vi "Q2_TorresHan.vi"() -> ()   [LabVIEW 2020]
uses:
  <vilib>/Utility/miscctls.llb/LVPoint32TypeDef.ctl
  <vilib>/Utility/miscctls.llb/LVPositionTypeDef.ctl
  <vilib>/Utility/miscctls.llb/LVBoundsTypeDef.ctl
  <vilib>/Utility/inputDevices.llb/mouseAcquire.vi
  <vilib>/Utility/inputDevices.llb/closeMouse.vi
panel:
  in  "instrucciones":bool
  out "pasos":string
  out "mensaje":string
  in  "Iniciar":bool
  out "estado":u16
  out "discoaMover":string
  out "positionIncialTorre":i32
  out "evento":u32
  out "positionIncialDisco":T1
  out "referenciaDisco":refnum<vi>
  out "mouseActivoPorEvento?":bool=TRUE
  out "mouse":bool
  out "coordenadas del mouse":T2
  out "Tu numero de movimientos":i16
  out "Minimos de movimientos":u16
  in  "Numero de discos":enum16{"3", "4", "5"}(ring)
  out "5":bool
  out "4":bool
  out "3":bool
  out "2":bool
  out "1":bool
  out "disco5 4":bool
  out "disco5 3":bool
  out "disco5 2":bool
  out "BASE":bool
  out "TORRE2":bool
  out "TORRE3":bool
  out "TORRE1":bool
  # "TORRE 1"
  # "TORRE 2"
  # "TORRE 3"
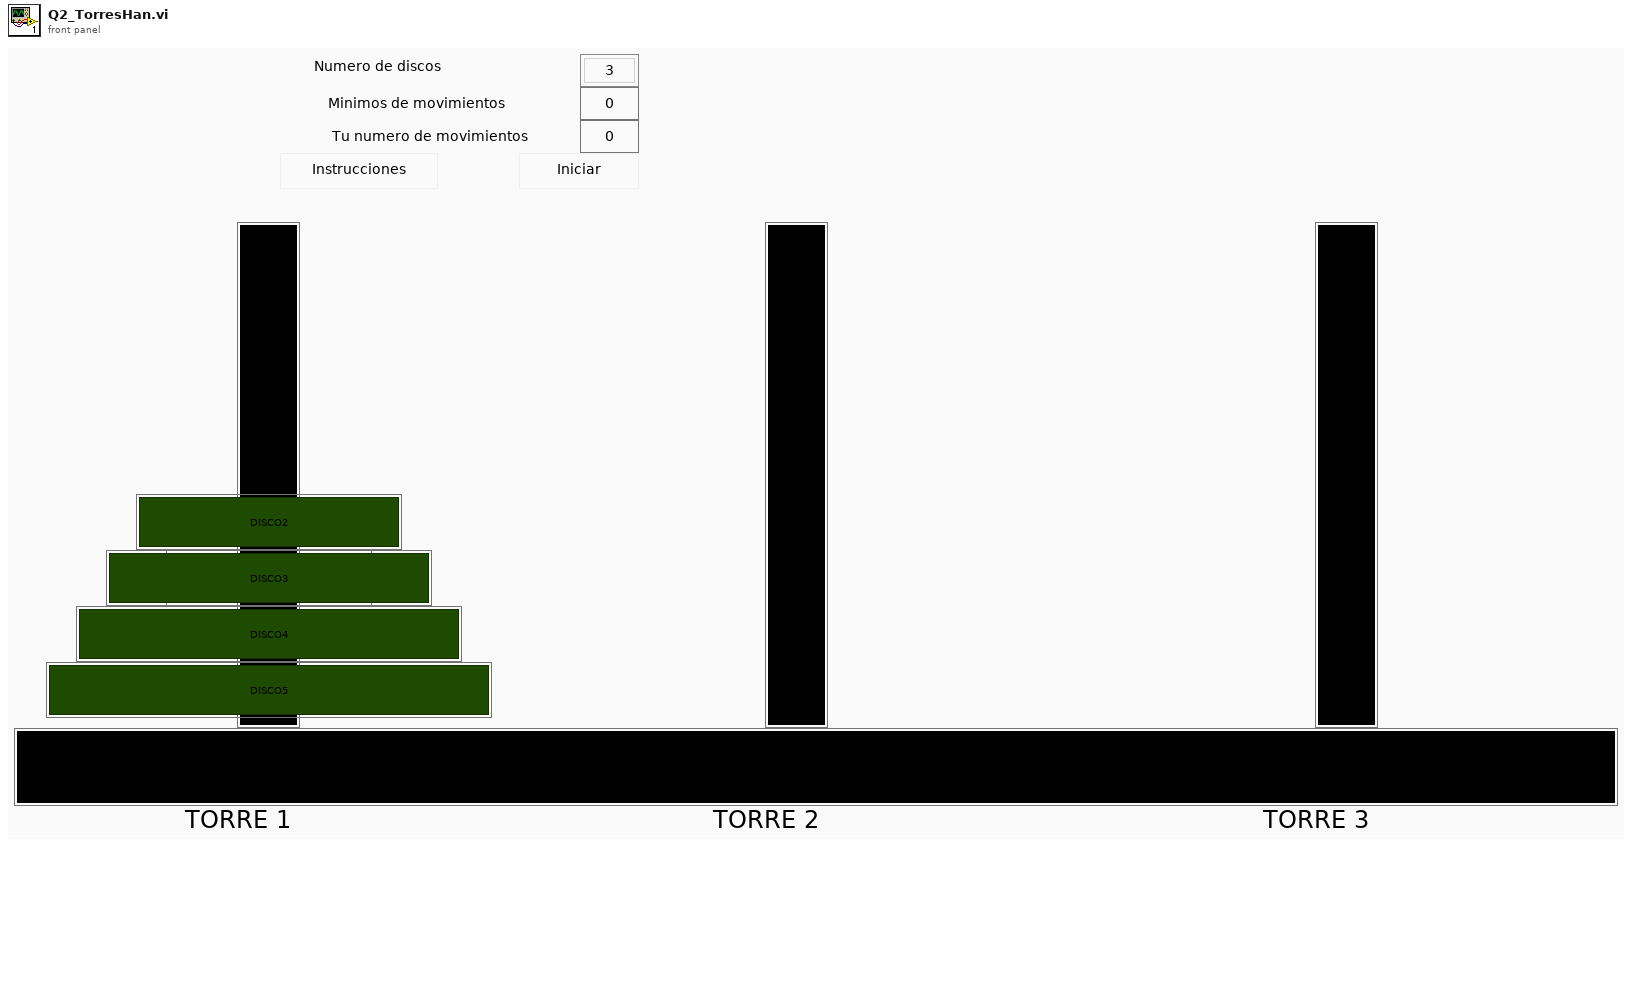
[diagram p1: front panel]
types:
  T1 = typedef "LVPositionTypeDef.ctl" = cluster{"Left":i32, "Top":i32}
  T2 = typedef "LVPoint32TypeDef.ctl" = cluster{"Horizontal":i32, "Vertical":i32}
  T3 = typedef "LVBoundsTypeDef.ctl" = cluster{"Width":u32, "Height":u32}
  T4 = cluster{"button 1":bool, "button 2":bool, "button 3":bool, "button 4":bool}
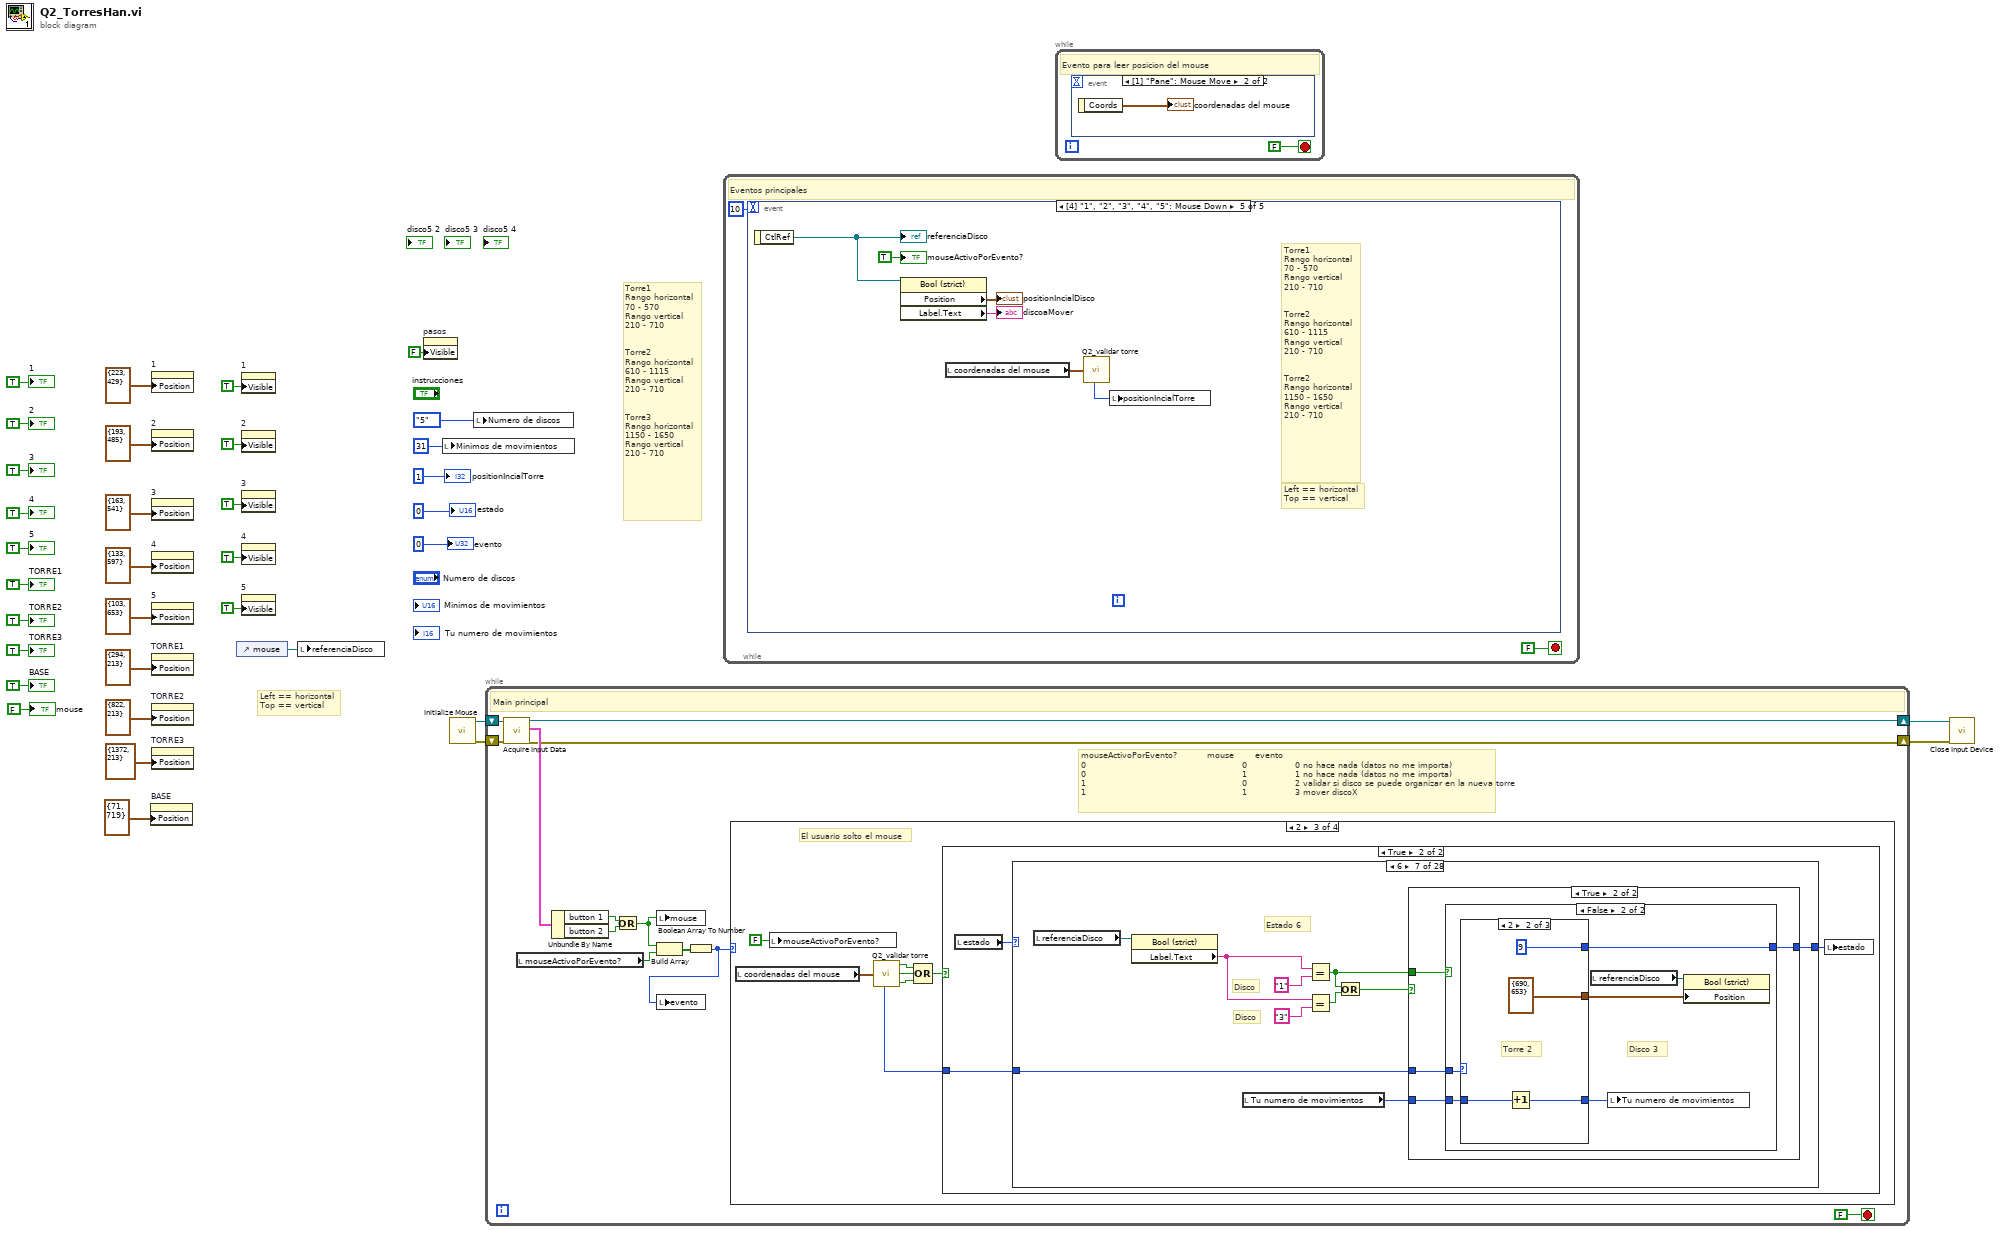
[diagram p0: block diagram]
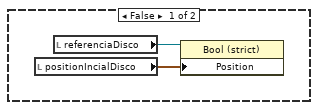
[diagram p4: hidden frame]
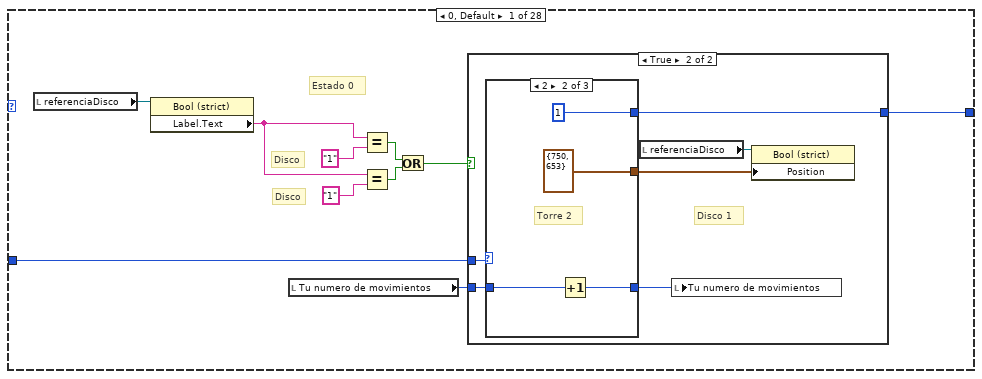
[diagram p5: hidden frame]
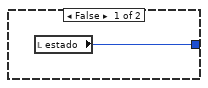
[diagram p6: hidden frame]
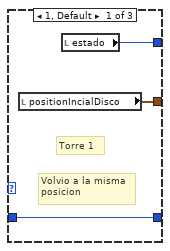
[diagram p7: hidden frame]
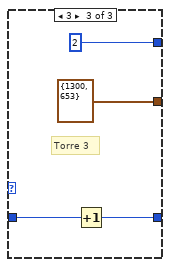
[diagram p8: hidden frame]
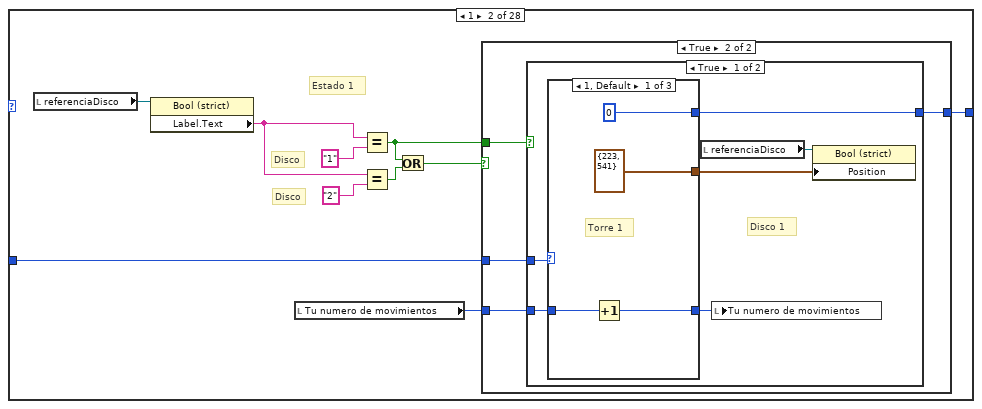
[diagram p9: hidden frame]
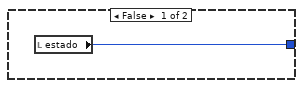
[diagram p10: hidden frame]
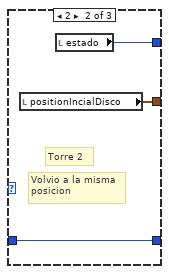
[diagram p11: hidden frame]
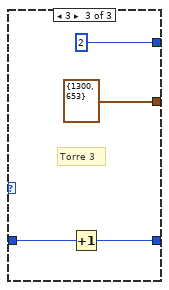
[diagram p12: hidden frame]
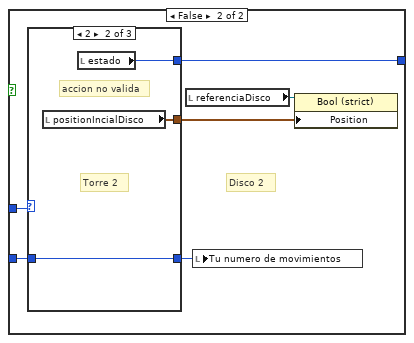
[diagram p13: hidden frame]
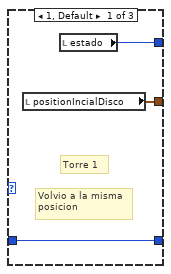
[diagram p14: hidden frame]
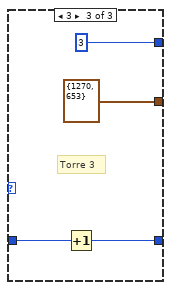
[diagram p15: hidden frame]
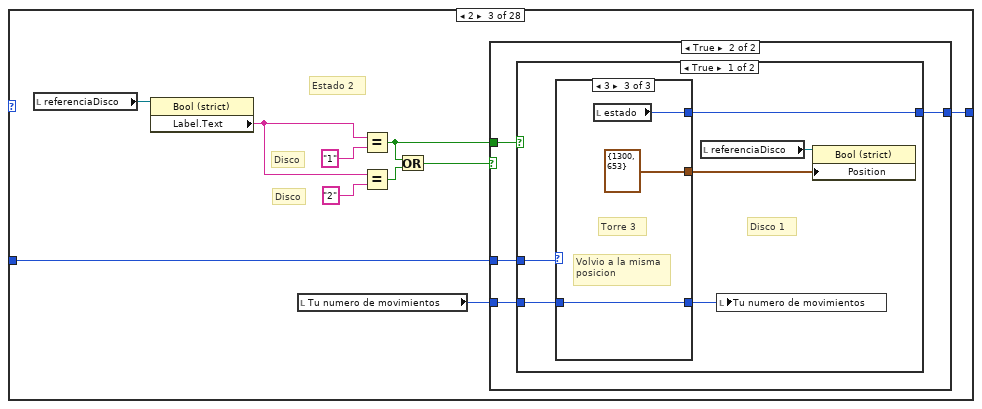
[diagram p16: hidden frame]
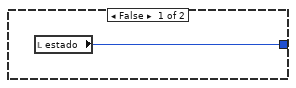
[diagram p17: hidden frame]
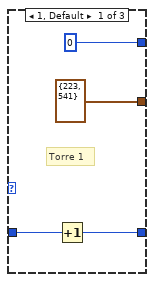
[diagram p18: hidden frame]
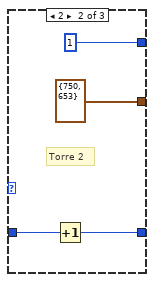
[diagram p19: hidden frame]
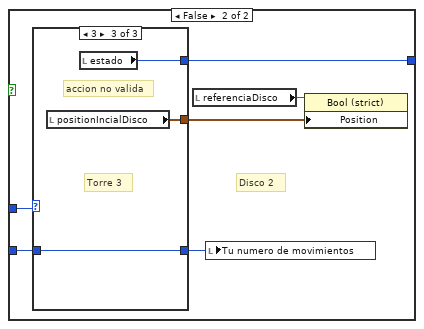
[diagram p20: hidden frame]
diagram:
  # "Left == horizontal\nTop == vertical"
  # "Torre1\nRango horizontal\n70 - 570\nRango vertical\n210 - 710\n\n\nTorre2\nRango horizontal\n610 - 1115\nRango vertical\n210 - 710\n\n\nTorre3\nRango horizontal\n1150 - 1650\nRango vertical\n210 - 710"
  n1 = property on="BASE" class="Bool (strict)"("Position"=T1 {"Left"=71, "Top"=719}) -> ()  [unwired: 2 in, 2 out]
  n2 = property on="1" class="Bool (strict)"("Position"=T1 {"Left"=223, "Top"=429}) -> ()  [unwired: 2 in, 2 out]
  n3 = property on="2" class="Bool (strict)"("Position"=T1 {"Left"=193, "Top"=485}) -> ()  [unwired: 2 in, 2 out]
  n4 = property on="3" class="Bool (strict)"("Position"=T1 {"Left"=163, "Top"=541}) -> ()  [unwired: 2 in, 2 out]
  n5 = property on="4" class="Bool (strict)"("Position"=T1 {"Left"=133, "Top"=597}) -> ()  [unwired: 2 in, 2 out]
  n6 = property on="5" class="Bool (strict)"("Position"=T1 {"Left"=103, "Top"=653}) -> ()  [unwired: 2 in, 2 out]
  n7 = property on="TORRE1" class="Bool (strict)"("Position"=T1 {"Left"=294, "Top"=213}) -> ()  [unwired: 2 in, 2 out]
  n8 = property on="TORRE2" class="Bool (strict)"("Position"=T1 {"Left"=822, "Top"=213}) -> ()  [unwired: 2 in, 2 out]
  n9 = property on="TORRE3" class="Bool (strict)"("Position"=T1 {"Left"=1372, "Top"=213}) -> ()  [unwired: 2 in, 2 out]
  n10 = control-ref of="mouse"() -> (w2:refnum<vi>)
  n11 = property on="1" class="Bool (strict)"("Visible"=TRUE) -> ()  [unwired: 2 in, 2 out]
  n12 = property on="2" class="Bool (strict)"("Visible"=TRUE) -> ()  [unwired: 2 in, 2 out]
  n13 = property on="3" class="Bool (strict)"("Visible"=TRUE) -> ()  [unwired: 2 in, 2 out]
  n14 = property on="4" class="Bool (strict)"("Visible"=TRUE) -> ()  [unwired: 2 in, 2 out]
  n15 = property on="5" class="Bool (strict)"("Visible"=TRUE) -> ()  [unwired: 2 in, 2 out]
  n16 = local write "referenciaDisco"(w2) -> ()
  n17 = property on="pasos" class="Str"("Visible"=FALSE) -> ()  [unwired: 2 in, 2 out]
  n18 = local write "Minimos de movimientos"(u16 31 ("Minimos de movimientos")) -> ()
  n19 = call <vilib>:"Initialize Mouse.vi"() -> ("error out"=w5:errorcluster, "device ID"=w6:refnum<k1>)  [unwired: 10 in]
  n20 = local write "Numero de discos"(enum16{"3", "4", "5"}."5" ("Numero de discos")) -> ()
  n21 = while {
    shift-right: [w44] -> w4
    shift-left: w6 -> [w46]
    shift-right: [w43] -> w3
    shift-left: w5 -> [w45]
    stop <- FALSE stop-if-true
    # "mouseActivoPorEvento?\t         mouse\t      evento\n0\t\t                                                  0\t               0 no hace nada (datos no me importa)\n0\t\t                                                  1\t               1 no hace nada (datos no me importa)\n1\t\t                                                  0\t               2 validar si disco se puede organizar en la nueva torre\n1\t\t                                                  1\t               3 mover discoX"
    # "Main principal"
    n22 = call-poly <vilib>:"Acquire Input Data.vi"("device ID"=w46, "error in (no error)"=w45) -> ("device ID"=w44:refnum<k1>, "button info"=w47:T4, "error out"=w43:errorcluster)  [unwired: 14 in, 1 out]
    n23 = local read "mouseActivoPorEvento?"() -> (w40:bool)
    n24 = Unbundle By Name(w47) -> ("button 1"=w42:bool, "button 2"=w41:bool)
    n25 = Or(x=w42, y=w41) -> (x .or. y?=w38:bool)
    n26 = local write "mouse"(w38) -> ()
    n27 = Build Array(w38, w40) -> (w39:bool[])
    n28 = Boolean Array To Number(Boolean array=w39) -> (number=w37:u32)
    n29 = local write "evento"(w37) -> ()
    n30 = case shown="2" w37 {
      frame 0, Default {
      }
      frame 1 {
      }
      frame 2 {
        # "El usuario solto el mouse"
        n31 = local read "coordenadas del mouse"() -> (w54:T2)
        n32 = local write "mouseActivoPorEvento?"(FALSE ("mouseActivoPorEvento?")) -> ()
        n33 = call "Q2_validar torre.vi"("coordenadas del mouse"=w54) -> ("Torre"=w48:i32, "torre1"=w51:bool, "torre2"=w52:bool, "torre3"=w53:bool)  [unwired: 3 in]
        n34 = Compound Arithmetic op=OR(w51, w52, w53) -> (w49:bool)
        n35 = case shown="True" w49 {
          tunnel: w48 -> [_ w59]
          frame False {
            n36 = local read "positionIncialDisco"() -> (w56:T1)
            n37 = local read "referenciaDisco"() -> (w55:refnum<vi>)
            n38 = property class="Bool (strict)"(reference=w55, "Position"=w56) -> ()  [unwired: 1 in, 2 out]
          }
          frame True {
            n39 = local read "estado"() -> (w58:u16)
            n40 = case shown="6" w58 {
              tunnel: w59 -> [w69 w97 w145 w193 w241 w289 w337 w385 w433 w481 w529 w577 w625 w673 w721 w769 w817 w865 w913 w961 w1009 w1037 w1085 w1133 w1181 w1229 w1257 w1305]
              tunnel: [w68 w96 w144 w192 w240 w288 w336 w384 w432 w480 w528 w576 w624 w672 w720 w768 w816 w864 w912 w960 w1008 w1036 w1084 w1132 w1180 w1228 w1256 w1304] -> w57
              frame 0, Default {
                # "Disco"
                # "Disco"
                # "Estado 0"
                n41 = local read "referenciaDisco"() -> (w64:refnum<vi>)
                n42 = property class="Bool (strict)"(reference=w64) -> ("Label.Text"=w65:string)  [unwired: 1 in, 2 out]
                n43 = local read "Tu numero de movimientos"() -> (w60:i16)
                n44 = Equal?(x=w65, y="1") -> (x = y?=w67:bool)
                n45 = Equal?(x=w65, y="1") -> (x = y?=w66:bool)
                n46 = Or(x=w67, y=w66) -> (x .or. y?=w61:bool)
                n47 = case shown="True" w61 {
                  tunnel: w69 -> [_ w75]
                  tunnel: [w70 w73] -> w68
                  tunnel: w60 -> [_ w71]
                  frame False {
                    n48 = local read "estado"() -> (w70:u16)
                  }
                  frame True {
                    # "Disco 1"
                    n49 = case shown="2" w75 {
                      tunnel: [w79 T1 {"Left"=750, "Top"=653} ("Position") T1 {"Left"=1300, "Top"=653} ("Position")] -> w74
                      tunnel: [w77 u16 1 ("estado") u16 2 ("estado")] -> w73
                      tunnel: [w78 w80 w84] -> w72
                      tunnel: w71 -> [w78 w81 w85]
                      frame 1, Default {
                        # "Volvio a la misma\nposicion"
                        # "Torre 1"
                        n50 = local read "positionIncialDisco"() -> (w79:T1)
                        n51 = local read "estado"() -> (w77:u16)
                      }
                      frame 2 {
                        # "Torre 2"
                        n52 = Increment(x=w81) -> (x+1=w80:i16)
                      }
                      frame 3 {
                        # "Torre 3"
                        n53 = Increment(x=w85) -> (x+1=w84:i16)
                      }
                    }
                    n54 = local read "referenciaDisco"() -> (w76:refnum<vi>)
                    n55 = local write "Tu numero de movimientos"(w72) -> ()
                    n56 = property class="Bool (strict)"(reference=w76, "Position"=w74) -> ()  [unwired: 1 in, 2 out]
                  }
                }
              }
              frame 1 {
                # "Disco"
                # "Disco"
                # "Estado 1"
                n57 = local read "referenciaDisco"() -> (w93:refnum<vi>)
                n58 = property class="Bool (strict)"(reference=w93) -> ("Label.Text"=w94:string)  [unwired: 1 in, 2 out]
                n59 = local read "Tu numero de movimientos"() -> (w88:i16)
                n60 = Equal?(x=w94, y="1") -> (x = y?=w89:bool)
                n61 = Equal?(x=w94, y="2") -> (x = y?=w95:bool)
                n62 = Or(x=w89, y=w95) -> (x .or. y?=w90:bool)
                n63 = case shown="True" w90 {
                  tunnel: w97 -> [_ w102]
                  tunnel: [w98 w101] -> w96
                  tunnel: w89 -> [_ w100]
                  tunnel: w88 -> [_ w99]
                  frame False {
                    n64 = local read "estado"() -> (w98:u16)
                  }
                  frame True {
                    n65 = case shown="True" w100 {
                      tunnel: w102 -> [w107 w124]
                      tunnel: [w105 w122] -> w101
                      tunnel: w99 -> [w103 w120]
                      frame True {
                        # "Disco 1"
                        n66 = case shown="1, Default" w107 {
                          tunnel: [T1 {"Left"=223, "Top"=541} ("Position") w114 T1 {"Left"=1300, "Top"=653} ("Position")] -> w106
                          tunnel: [u16 0 ("estado") w113 u16 2 ("estado")] -> w105
                          tunnel: [w109 w115 w116] -> w104
                          tunnel: w103 -> [w110 w115 w117]
                          frame 1, Default {
                            # "Torre 1"
                            n67 = Increment(x=w110) -> (x+1=w109:i16)
                          }
                          frame 2 {
                            # "Volvio a la misma\nposicion"
                            # "Torre 2"
                            n68 = local read "positionIncialDisco"() -> (w114:T1)
                            n69 = local read "estado"() -> (w113:u16)
                          }
                          frame 3 {
                            # "Torre 3"
                            n70 = Increment(x=w117) -> (x+1=w116:i16)
                          }
                        }
                        n71 = local read "referenciaDisco"() -> (w108:refnum<vi>)
                        n72 = local write "Tu numero de movimientos"(w104) -> ()
                        n73 = property class="Bool (strict)"(reference=w108, "Position"=w106) -> ()  [unwired: 1 in, 2 out]
                      }
                      frame False {
                        # "Disco 2"
                        n74 = case shown="2" w124 {
                          tunnel: [w128 w131 T1 {"Left"=1270, "Top"=653} ("Position")] -> w123
                          tunnel: [w126 w129 u16 3 ("estado")] -> w122
                          tunnel: [w127 w130 w132] -> w121
                          tunnel: w120 -> [w127 w130 w133]
                          frame 1, Default {
                            # "Volvio a la misma\nposicion"
                            # "Torre 1"
                            n75 = local read "positionIncialDisco"() -> (w128:T1)
                            n76 = local read "estado"() -> (w126:u16)
                          }
                          frame 2 {
                            # "accion no valida"
                            # "Torre 2"
                            n77 = local read "positionIncialDisco"() -> (w131:T1)
                            n78 = local read "estado"() -> (w129:u16)
                          }
                          frame 3 {
                            # "Torre 3"
                            n79 = Increment(x=w133) -> (x+1=w132:i16)
                          }
                        }
                        n80 = local read "referenciaDisco"() -> (w125:refnum<vi>)
                        n81 = local write "Tu numero de movimientos"(w121) -> ()
                        n82 = property class="Bool (strict)"(reference=w125, "Position"=w123) -> ()  [unwired: 1 in, 2 out]
                      }
                    }
                  }
                }
              }
              frame 2 {
                # "Disco"
                # "Disco"
                # "Estado 2"
                n83 = local read "referenciaDisco"() -> (w141:refnum<vi>)
                n84 = property class="Bool (strict)"(reference=w141) -> ("Label.Text"=w142:string)  [unwired: 1 in, 2 out]
                n85 = local read "Tu numero de movimientos"() -> (w136:i16)
                n86 = Equal?(x=w142, y="1") -> (x = y?=w137:bool)
                n87 = Equal?(x=w142, y="2") -> (x = y?=w143:bool)
                n88 = Or(x=w137, y=w143) -> (x .or. y?=w138:bool)
                n89 = case shown="True" w138 {
                  tunnel: w145 -> [_ w150]
                  tunnel: [w146 w149] -> w144
                  tunnel: w137 -> [_ w148]
                  tunnel: w136 -> [_ w147]
                  frame False {
                    n90 = local read "estado"() -> (w146:u16)
                  }
                  frame True {
                    n91 = case shown="True" w148 {
                      tunnel: w150 -> [w155 w172]
                      tunnel: [w153 w170] -> w149
                      tunnel: w147 -> [w151 w168]
                      frame True {
                        # "Disco 1"
                        n92 = case shown="3" w155 {
                          tunnel: [T1 {"Left"=223, "Top"=541} ("Position") T1 {"Left"=750, "Top"=653} ("Position") T1 {"Left"=1300, "Top"=653} ("Position")] -> w154
                          tunnel: [u16 0 ("estado") u16 1 ("estado") w165] -> w153
                          tunnel: [w157 w161 w166] -> w152
                          tunnel: w151 -> [w158 w162 w166]
                          frame 1, Default {
                            # "Torre 1"
                            n93 = Increment(x=w158) -> (x+1=w157:i16)
                          }
                          frame 2 {
                            # "Torre 2"
                            n94 = Increment(x=w162) -> (x+1=w161:i16)
                          }
                          frame 3 {
                            # "Volvio a la misma\nposicion"
                            # "Torre 3"
                            n95 = local read "estado"() -> (w165:u16)
                          }
                        }
                        n96 = local read "referenciaDisco"() -> (w156:refnum<vi>)
                        n97 = local write "Tu numero de movimientos"(w152) -> ()
                        n98 = property class="Bool (strict)"(reference=w156, "Position"=w154) -> ()  [unwired: 1 in, 2 out]
                      }
                      frame False {
                        # "Disco 2"
                        n99 = case shown="3" w172 {
                          tunnel: [w176 T1 {"Left"=720, "Top"=653} ("Position") w183] -> w171
                          tunnel: [w174 u16 4 ("estado") w181] -> w170
                          tunnel: [w175 w177 w182] -> w169
                          tunnel: w168 -> [w175 w178 w182]
                          frame 1, Default {
                            # "Volvio a la misma\nposicion"
                            # "Torre 1"
                            n100 = local read "positionIncialDisco"() -> (w176:T1)
                            n101 = local read "estado"() -> (w174:u16)
                          }
                          frame 2 {
                            # "Torre 2"
                            n102 = Increment(x=w178) -> (x+1=w177:i16)
                          }
                          frame 3 {
                            # "accion no valida"
                            # "Torre 3"
                            n103 = local read "positionIncialDisco"() -> (w183:T1)
                            n104 = local read "estado"() -> (w181:u16)
                          }
                        }
                        n105 = local read "referenciaDisco"() -> (w173:refnum<vi>)
                        n106 = local write "Tu numero de movimientos"(w169) -> ()
                        n107 = property class="Bool (strict)"(reference=w173, "Position"=w171) -> ()  [unwired: 1 in, 2 out]
                      }
                    }
                  }
                }
              }
              frame 3 {
                # "Disco"
                # "Disco"
                # "Estado 3"
                n108 = local read "referenciaDisco"() -> (w189:refnum<vi>)
                n109 = property class="Bool (strict)"(reference=w189) -> ("Label.Text"=w190:string)  [unwired: 1 in, 2 out]
                n110 = local read "Tu numero de movimientos"() -> (w184:i16)
                n111 = Equal?(x=w190, y="1") -> (x = y?=w185:bool)
                n112 = Equal?(x=w190, y="2") -> (x = y?=w191:bool)
                n113 = Or(x=w185, y=w191) -> (x .or. y?=w186:bool)
                n114 = case shown="True" w186 {
                  tunnel: w193 -> [_ w198]
                  tunnel: [w194 w197] -> w192
                  tunnel: w185 -> [_ w196]
                  tunnel: w184 -> [_ w195]
                  frame False {
                    n115 = local read "estado"() -> (w194:u16)
                  }
                  frame True {
                    n116 = case shown="True" w196 {
                      tunnel: w198 -> [w203 w220]
                      tunnel: [w201 w218] -> w197
                      tunnel: w195 -> [w199 w216]
                      frame True {
                        # "Disco 1"
                        n117 = case shown="3" w203 {
                          tunnel: [T1 {"Left"=223, "Top"=597} ("Position") w211 T1 {"Left"=1300, "Top"=597} ("Position")] -> w202
                          tunnel: [u16 5 ("estado") w210 u16 6 ("estado")] -> w201
                          tunnel: [w205 w209 w212] -> w200
                          tunnel: w199 -> [w206 w209 w213]
                          frame 1, Default {
                            # "Torre 1"
                            n118 = Increment(x=w206) -> (x+1=w205:i16)
                          }
                          frame 2 {
                            # "Volvio a la misma\nposicion"
                            # "Torre 2"
                            n119 = local read "positionIncialDisco"() -> (w211:T1)
                            n120 = local read "estado"() -> (w210:u16)
                          }
                          frame 3 {
                            # "Torre 3"
                            n121 = Increment(x=w213) -> (x+1=w212:i16)
                          }
                        }
                        n122 = local read "referenciaDisco"() -> (w204:refnum<vi>)
                        n123 = local write "Tu numero de movimientos"(w200) -> ()
                        n124 = property class="Bool (strict)"(reference=w204, "Position"=w202) -> ()  [unwired: 1 in, 2 out]
                      }
                      frame False {
                        # "Disco 2"
                        n125 = case shown="2" w220 {
                          tunnel: [T1 {"Left"=193, "Top"=597} ("Position") w228 w231] -> w219
                          tunnel: [u16 1 ("estado") w226 w230] -> w218
                          tunnel: [w222 w227 w229] -> w217
                          tunnel: w216 -> [w223 w227 w229]
                          frame 1, Default {
                            # "Torre 1"
                            n126 = Increment(x=w223) -> (x+1=w222:i16)
                          }
                          frame 2 {
                            # "accion no valida"
                            # "Torre 2"
                            n127 = local read "positionIncialDisco"() -> (w228:T1)
                            n128 = local read "estado"() -> (w226:u16)
                          }
                          frame 3 {
                            # "Volvio a la misma\nposicion"
                            # "Torre 3"
                            n129 = local read "positionIncialDisco"() -> (w231:T1)
                            n130 = local read "estado"() -> (w230:u16)
                          }
                        }
                        n131 = local read "referenciaDisco"() -> (w221:refnum<vi>)
                        n132 = local write "Tu numero de movimientos"(w217) -> ()
                        n133 = property class="Bool (strict)"(reference=w221, "Position"=w219) -> ()  [unwired: 1 in, 2 out]
                      }
                    }
                  }
                }
              }
              frame 4 {
                # "Disco"
                # "Disco"
                # "Estado 4"
                n134 = local read "referenciaDisco"() -> (w237:refnum<vi>)
                n135 = property class="Bool (strict)"(reference=w237) -> ("Label.Text"=w238:string)  [unwired: 1 in, 2 out]
                n136 = local read "Tu numero de movimientos"() -> (w232:i16)
                n137 = Equal?(x=w238, y="1") -> (x = y?=w233:bool)
                n138 = Equal?(x=w238, y="2") -> (x = y?=w239:bool)
                n139 = Or(x=w233, y=w239) -> (x .or. y?=w234:bool)
                n140 = case shown="True" w234 {
                  tunnel: w241 -> [_ w246]
                  tunnel: [w242 w245] -> w240
                  tunnel: w233 -> [_ w244]
                  tunnel: w232 -> [_ w243]
                  frame False {
                    n141 = local read "estado"() -> (w242:u16)
                  }
                  frame True {
                    n142 = case shown="True" w244 {
                      tunnel: w246 -> [w251 w268]
                      tunnel: [w249 w266] -> w245
                      tunnel: w243 -> [w247 w264]
                      frame True {
                        # "Disco 1"
                        n143 = case shown="2" w251 {
                          tunnel: [T1 {"Left"=223, "Top"=597} ("Position") T1 {"Left"=750, "Top"=597} ("Position") w263] -> w250
                          tunnel: [u16 7 ("estado") u16 8 ("estado") w262] -> w249
                          tunnel: [w253 w257 w261] -> w248
                          tunnel: w247 -> [w254 w258 w261]
                          frame 1, Default {
                            # "Torre 1"
                            n144 = Increment(x=w254) -> (x+1=w253:i16)
                          }
                          frame 2 {
                            # "Torre 2"
                            n145 = Increment(x=w258) -> (x+1=w257:i16)
                          }
                          frame 3 {
                            # "Volvio a la misma\nposicion"
                            # "Torre 3"
                            n146 = local read "positionIncialDisco"() -> (w263:T1)
                            n147 = local read "estado"() -> (w262:u16)
                          }
                        }
                        n148 = local read "referenciaDisco"() -> (w252:refnum<vi>)
                        n149 = local write "Tu numero de movimientos"(w248) -> ()
                        n150 = property class="Bool (strict)"(reference=w252, "Position"=w250) -> ()  [unwired: 1 in, 2 out]
                      }
                      frame False {
                        # "Disco 2"
                        n151 = case shown="3" w268 {
                          tunnel: [T1 {"Left"=193, "Top"=597} ("Position") w276 w279] -> w267
                          tunnel: [u16 2 ("estado") w274 w277] -> w266
                          tunnel: [w270 w275 w278] -> w265
                          tunnel: w264 -> [w271 w275 w278]
                          frame 1, Default {
                            # "Torre 1"
                            n152 = Increment(x=w271) -> (x+1=w270:i16)
                          }
                          frame 2 {
                            # "Volvio a la misma\nposicion"
                            # "Torre 2"
                            n153 = local read "positionIncialDisco"() -> (w276:T1)
                            n154 = local read "estado"() -> (w274:u16)
                          }
                          frame 3 {
                            # "accion no valida"
                            # "Torre 3"
                            n155 = local read "positionIncialDisco"() -> (w279:T1)
                            n156 = local read "estado"() -> (w277:u16)
                          }
                        }
                        n157 = local read "referenciaDisco"() -> (w269:refnum<vi>)
                        n158 = local write "Tu numero de movimientos"(w265) -> ()
                        n159 = property class="Bool (strict)"(reference=w269, "Position"=w267) -> ()  [unwired: 1 in, 2 out]
                      }
                    }
                  }
                }
              }
              frame 5 {
                # "Disco"
                # "Disco"
                # "Estado 5"
                n160 = local read "referenciaDisco"() -> (w285:refnum<vi>)
                n161 = property class="Bool (strict)"(reference=w285) -> ("Label.Text"=w286:string)  [unwired: 1 in, 2 out]
                n162 = local read "Tu numero de movimientos"() -> (w280:i16)
                n163 = Equal?(x=w286, y="1") -> (x = y?=w281:bool)
                n164 = Equal?(x=w286, y="2") -> (x = y?=w287:bool)
                n165 = Or(x=w281, y=w287) -> (x .or. y?=w282:bool)
                n166 = case shown="True" w282 {
                  tunnel: w289 -> [_ w294]
                  tunnel: [w290 w293] -> w288
                  tunnel: w281 -> [_ w292]
                  tunnel: w280 -> [_ w291]
                  frame False {
                    n167 = local read "estado"() -> (w290:u16)
                  }
                  frame True {
                    n168 = case shown="False" w292 {
                      tunnel: w294 -> [w299 w316]
                      tunnel: [w297 w314] -> w293
                      tunnel: w291 -> [w295 w312]
                      frame True {
                        # "Disco 1"
                        n169 = case shown="1, Default" w299 {
                          tunnel: [w301 T1 {"Left"=750, "Top"=653} ("Position") T1 {"Left"=1300, "Top"=597} ("Position")] -> w298
                          tunnel: [w302 u16 3 ("estado") u16 6 ("estado")] -> w297
                          tunnel: [w303 w304 w308] -> w296
                          tunnel: w295 -> [w303 w305 w311]
                          frame 1, Default {
                            # "Volvio a la misma\nposicion"
                            # "Torre 1"
                            n170 = local read "positionIncialDisco"() -> (w301:T1)
                            n171 = local read "estado"() -> (w302:u16)
                          }
                          frame 2 {
                            # "Torre 2"
                            n172 = Increment(x=w305) -> (x+1=w304:i16)
                          }
                          frame 3 {
                            # "Torre 3"
                            n173 = Increment(x=w311) -> (x+1=w308:i16)
                          }
                        }
                        n174 = local read "referenciaDisco"() -> (w300:refnum<vi>)
                        n175 = local write "Tu numero de movimientos"(w296) -> ()
                        n176 = property class="Bool (strict)"(reference=w300, "Position"=w298) -> ()  [unwired: 1 in, 2 out]
                      }
                      frame False {
                        # "Disco 2"
                        n177 = case shown="1, Default" w316 {
                          tunnel: [w319 T1 {"Left"=720, "Top"=653} ("Position") w326] -> w315
                          tunnel: [w318 u16 7 ("estado") w325] -> w314
                          tunnel: [w320 w322 w327] -> w313
                          tunnel: w312 -> [w320 w324 w327]
                          frame 1, Default {
                            # "accion no valida"
                            # "Torre 1"
                            n178 = local read "positionIncialDisco"() -> (w319:T1)
                            n179 = local read "estado"() -> (w318:u16)
                          }
                          frame 2 {
                            # "Torre 2"
                            n180 = Increment(x=w324) -> (x+1=w322:i16)
                          }
                          frame 3 {
                            # "Volvio a la misma\nposicion"
                            # "Torre 3"
                            n181 = local read "positionIncialDisco"() -> (w326:T1)
                            n182 = local read "estado"() -> (w325:u16)
                          }
                        }
                        n183 = local read "referenciaDisco"() -> (w317:refnum<vi>)
                        n184 = local write "Tu numero de movimientos"(w313) -> ()
                        n185 = property class="Bool (strict)"(reference=w317, "Position"=w315) -> ()  [unwired: 1 in, 2 out]
                      }
                    }
                  }
                }
              }
              frame 6 {
                # "Disco"
                # "Disco"
                # "Estado 6"
                n186 = local read "referenciaDisco"() -> (w333:refnum<vi>)
                n187 = property class="Bool (strict)"(reference=w333) -> ("Label.Text"=w334:string)  [unwired: 1 in, 2 out]
                n188 = local read "Tu numero de movimientos"() -> (w328:i16)
                n189 = Equal?(x=w334, y="1") -> (x = y?=w329:bool)
                n190 = Equal?(x=w334, y="3") -> (x = y?=w335:bool)
                n191 = Or(x=w329, y=w335) -> (x .or. y?=w330:bool)
                n192 = case shown="True" w330 {
                  tunnel: w337 -> [_ w342]
                  tunnel: [w338 w341] -> w336
                  tunnel: w329 -> [_ w340]
                  tunnel: w328 -> [_ w339]
                  frame False {
                    n193 = local read "estado"() -> (w338:u16)
                  }
                  frame True {
                    n194 = case shown="False" w340 {
                      tunnel: w342 -> [w347 w364]
                      tunnel: [w345 w362] -> w341
                      tunnel: w339 -> [w343 w360]
                      frame True {
                        # "Disco 1"
                        n195 = case shown="1, Default" w347 {
                          tunnel: [T1 {"Left"=223, "Top"=597} ("Position") T1 {"Left"=750, "Top"=653} ("Position") w357] -> w346
                          tunnel: [u16 5 ("estado") u16 3 ("estado") w358] -> w345
                          tunnel: [w349 w353 w359] -> w344
                          tunnel: w343 -> [w352 w354 w359]
                          frame 1, Default {
                            # "Torre 1"
                            n196 = Increment(x=w352) -> (x+1=w349:i16)
                          }
                          frame 2 {
                            # "Torre 2"
                            n197 = Increment(x=w354) -> (x+1=w353:i16)
                          }
                          frame 3 {
                            # "Volvio a la misma\nposicion"
                            # "Torre 3"
                            n198 = local read "positionIncialDisco"() -> (w357:T1)
                            n199 = local read "estado"() -> (w358:u16)
                          }
                        }
                        n200 = local read "referenciaDisco"() -> (w348:refnum<vi>)
                        n201 = local write "Tu numero de movimientos"(w344) -> ()
                        n202 = property class="Bool (strict)"(reference=w348, "Position"=w346) -> ()  [unwired: 1 in, 2 out]
                      }
                      frame False {
                        # "Disco 3"
                        n203 = case shown="2" w364 {
                          tunnel: [w367 T1 {"Left"=690, "Top"=653} ("Position") w374] -> w363
                          tunnel: [w366 u16 9 ("estado") w373] -> w362
                          tunnel: [w368 w370 w375] -> w361
                          tunnel: w360 -> [w368 w372 w375]
                          frame 1, Default {
                            # "Volvio a la misma\nposicion"
                            # "Torre 1"
                            n204 = local read "positionIncialDisco"() -> (w367:T1)
                            n205 = local read "estado"() -> (w366:u16)
                          }
                          frame 2 {
                            # "Torre 2"
                            n206 = Increment(x=w372) -> (x+1=w370:i16)
                          }
                          frame 3 {
                            # "accion no valida"
                            # "Torre 3"
                            n207 = local read "positionIncialDisco"() -> (w374:T1)
                            n208 = local read "estado"() -> (w373:u16)
                          }
                        }
                        n209 = local read "referenciaDisco"() -> (w365:refnum<vi>)
                        n210 = local write "Tu numero de movimientos"(w361) -> ()
                        n211 = property class="Bool (strict)"(reference=w365, "Position"=w363) -> ()  [unwired: 1 in, 2 out]
                      }
                    }
                  }
                }
              }
              frame 7 {
                # "Disco"
                # "Disco"
                # "Estado 7"
                n212 = local read "referenciaDisco"() -> (w381:refnum<vi>)
                n213 = property class="Bool (strict)"(reference=w381) -> ("Label.Text"=w382:string)  [unwired: 1 in, 2 out]
                n214 = local read "Tu numero de movimientos"() -> (w376:i16)
                n215 = Equal?(x=w382, y="1") -> (x = y?=w377:bool)
                n216 = Equal?(x=w382, y="2") -> (x = y?=w383:bool)
                n217 = Or(x=w377, y=w383) -> (x .or. y?=w378:bool)
                n218 = case shown="True" w378 {
                  tunnel: w385 -> [_ w390]
                  tunnel: [w386 w389] -> w384
                  tunnel: w377 -> [_ w388]
                  tunnel: w376 -> [_ w387]
                  frame False {
                    n219 = local read "estado"() -> (w386:u16)
                  }
                  frame True {
                    n220 = case shown="False" w388 {
                      tunnel: w390 -> [w395 w412]
                      tunnel: [w393 w410] -> w389
                      tunnel: w387 -> [w391 w408]
                      frame True {
                        # "Disco 1"
                        n221 = case shown="3" w395 {
                          tunnel: [w398 T1 {"Left"=750, "Top"=597} ("Position") T1 {"Left"=1300, "Top"=653} ("Position")] -> w394
                          tunnel: [w397 u16 8 ("estado") u16 4 ("estado")] -> w393
                          tunnel: [w399 w400 w405] -> w392
                          tunnel: w391 -> [w399 w401 w407]
                          frame 1, Default {
                            # "Volvio a la misma\nposicion"
                            # "Torre 1"
                            n222 = local read "positionIncialDisco"() -> (w398:T1)
                            n223 = local read "estado"() -> (w397:u16)
                          }
                          frame 2 {
                            # "Torre 2"
                            n224 = Increment(x=w401) -> (x+1=w400:i16)
                          }
                          frame 3 {
                            # "Torre 3"
                            n225 = Increment(x=w407) -> (x+1=w405:i16)
                          }
                        }
                        n226 = local read "referenciaDisco"() -> (w396:refnum<vi>)
                        n227 = local write "Tu numero de movimientos"(w392) -> ()
                        n228 = property class="Bool (strict)"(reference=w396, "Position"=w394) -> ()  [unwired: 1 in, 2 out]
                      }
                      frame False {
                        # "Disco 2"
                        n229 = case shown="3" w412 {
                          tunnel: [w415 w418 T1 {"Left"=1270, "Top"=653} ("Position")] -> w411
                          tunnel: [w414 w417 u16 5 ("estado")] -> w410
                          tunnel: [w416 w419 w421] -> w409
                          tunnel: w408 -> [w416 w419 w423]
                          frame 1, Default {
                            # "accion no valida"
                            # "Torre 1"
                            n230 = local read "positionIncialDisco"() -> (w415:T1)
                            n231 = local read "estado"() -> (w414:u16)
                          }
                          frame 2 {
                            # "Volvio a la misma\nposicion"
                            # "Torre 2"
                            n232 = local read "positionIncialDisco"() -> (w418:T1)
                            n233 = local read "estado"() -> (w417:u16)
                          }
                          frame 3 {
                            # "Torre 3"
                            n234 = Increment(x=w423) -> (x+1=w421:i16)
                          }
                        }
                        n235 = local read "referenciaDisco"() -> (w413:refnum<vi>)
                        n236 = local write "Tu numero de movimientos"(w409) -> ()
                        n237 = property class="Bool (strict)"(reference=w413, "Position"=w411) -> ()  [unwired: 1 in, 2 out]
                      }
                    }
                  }
                }
              }
              frame 8 {
                # "Disco"
                # "Disco"
                # "Estado 8"
                n238 = local read "referenciaDisco"() -> (w429:refnum<vi>)
                n239 = property class="Bool (strict)"(reference=w429) -> ("Label.Text"=w430:string)  [unwired: 1 in, 2 out]
                n240 = local read "Tu numero de movimientos"() -> (w424:i16)
                n241 = Equal?(x=w430, y="1") -> (x = y?=w425:bool)
                n242 = Equal?(x=w430, y="3") -> (x = y?=w431:bool)
                n243 = Or(x=w425, y=w431) -> (x .or. y?=w426:bool)
                n244 = case shown="True" w426 {
                  tunnel: w433 -> [_ w438]
                  tunnel: [w434 w437] -> w432
                  tunnel: w425 -> [_ w436]
                  tunnel: w424 -> [_ w435]
                  frame False {
                    n245 = local read "estado"() -> (w434:u16)
                  }
                  frame True {
                    n246 = case shown="False" w436 {
                      tunnel: w438 -> [w443 w460]
                      tunnel: [w441 w458] -> w437
                      tunnel: w435 -> [w439 w456]
                      frame True {
                        # "Disco 1"
                        n247 = case shown="3" w443 {
                          tunnel: [T1 {"Left"=223, "Top"=597} ("Position") w450 T1 {"Left"=1300, "Top"=653} ("Position")] -> w442
                          tunnel: [u16 7 ("estado") w449 u16 4 ("estado")] -> w441
                          tunnel: [w447 w451 w453] -> w440
                          tunnel: w439 -> [w448 w451 w455]
                          frame 1, Default {
                            # "Torre 1"
                            n248 = Increment(x=w448) -> (x+1=w447:i16)
                          }
                          frame 2 {
                            # "Volvio a la misma\nposicion"
                            # "Torre 2"
                            n249 = local read "positionIncialDisco"() -> (w450:T1)
                            n250 = local read "estado"() -> (w449:u16)
                          }
                          frame 3 {
                            # "Torre 3"
                            n251 = Increment(x=w455) -> (x+1=w453:i16)
                          }
                        }
                        n252 = local read "referenciaDisco"() -> (w444:refnum<vi>)
                        n253 = local write "Tu numero de movimientos"(w440) -> ()
                        n254 = property class="Bool (strict)"(reference=w444, "Position"=w442) -> ()  [unwired: 1 in, 2 out]
                      }
                      frame False {
                        # "Disco 3"
                        n255 = case shown="3" w460 {
                          tunnel: [w463 w466 T1 {"Left"=1240, "Top"=653} ("Position")] -> w459
                          tunnel: [w462 w465 u16 10 ("estado")] -> w458
                          tunnel: [w464 w467 w469] -> w457
                          tunnel: w456 -> [w464 w467 w471]
                          frame 1, Default {
                            # "Volvio a la misma\nposicion"
                            # "Torre 1"
                            n256 = local read "positionIncialDisco"() -> (w463:T1)
                            n257 = local read "estado"() -> (w462:u16)
                          }
                          frame 2 {
                            # "accion no valida"
                            # "Torre 2"
                            n258 = local read "positionIncialDisco"() -> (w466:T1)
                            n259 = local read "estado"() -> (w465:u16)
                          }
                          frame 3 {
                            # "Torre 3"
                            n260 = Increment(x=w471) -> (x+1=w469:i16)
                          }
                        }
                        n261 = local read "referenciaDisco"() -> (w461:refnum<vi>)
                        n262 = local write "Tu numero de movimientos"(w457) -> ()
                        n263 = property class="Bool (strict)"(reference=w461, "Position"=w459) -> ()  [unwired: 1 in, 2 out]
                      }
                    }
                  }
                }
              }
              frame 9 {
                # "Disco"
                # "Disco"
                # "Estado 9"
                n264 = local read "referenciaDisco"() -> (w477:refnum<vi>)
                n265 = property class="Bool (strict)"(reference=w477) -> ("Label.Text"=w478:string)  [unwired: 1 in, 2 out]
                n266 = local read "Tu numero de movimientos"() -> (w472:i16)
                n267 = Equal?(x=w478, y="1") -> (x = y?=w473:bool)
                n268 = Equal?(x=w478, y="3") -> (x = y?=w479:bool)
                n269 = Or(x=w473, y=w479) -> (x .or. y?=w474:bool)
                n270 = case shown="True" w474 {
                  tunnel: w481 -> [_ w486]
                  tunnel: [w482 w485] -> w480
                  tunnel: w473 -> [_ w484]
                  tunnel: w472 -> [_ w483]
                  frame False {
                    n271 = local read "estado"() -> (w482:u16)
                  }
                  frame True {
                    n272 = case shown="True" w484 {
                      tunnel: w486 -> [w491 w508]
                      tunnel: [w489 w506] -> w485
                      tunnel: w483 -> [w487 w504]
                      frame True {
                        # "Disco 1"
                        n273 = case shown="2" w491 {
                          tunnel: [T1 {"Left"=223, "Top"=653} ("Position") T1 {"Left"=750, "Top"=597} ("Position") w502] -> w490
                          tunnel: [u16 11 ("estado") u16 12 ("estado") w501] -> w489
                          tunnel: [w495 w497 w503] -> w488
                          tunnel: w487 -> [w496 w500 w503]
                          frame 1, Default {
                            # "Torre 1"
                            n274 = Increment(x=w496) -> (x+1=w495:i16)
                          }
                          frame 2 {
                            # "Torre 2"
                            n275 = Increment(x=w500) -> (x+1=w497:i16)
                          }
                          frame 3 {
                            # "Volvio a la misma\nposicion"
                            # "Torre 3"
                            n276 = local read "positionIncialDisco"() -> (w502:T1)
                            n277 = local read "estado"() -> (w501:u16)
                          }
                        }
                        n278 = local read "referenciaDisco"() -> (w492:refnum<vi>)
                        n279 = local write "Tu numero de movimientos"(w488) -> ()
                        n280 = property class="Bool (strict)"(reference=w492, "Position"=w490) -> ()  [unwired: 1 in, 2 out]
                      }
                      frame False {
                        # "Disco 3"
                        n281 = case shown="1, Default" w508 {
                          tunnel: [T1 {"Left"=163, "Top"=653} ("Position") w515 w518] -> w507
                          tunnel: [u16 6 ("estado") w514 w517] -> w506
                          tunnel: [w510 w516 w519] -> w505
                          tunnel: w504 -> [w513 w516 w519]
                          frame 1, Default {
                            # "Torre 1"
                            n282 = Increment(x=w513) -> (x+1=w510:i16)
                          }
                          frame 2 {
                            # "Volvio a la misma\nposicion"
                            # "Torre 2"
                            n283 = local read "positionIncialDisco"() -> (w515:T1)
                            n284 = local read "estado"() -> (w514:u16)
                          }
                          frame 3 {
                            # "accion no valida"
                            # "Torre 3"
                            n285 = local read "positionIncialDisco"() -> (w518:T1)
                            n286 = local read "estado"() -> (w517:u16)
                          }
                        }
                        n287 = local read "referenciaDisco"() -> (w509:refnum<vi>)
                        n288 = local write "Tu numero de movimientos"(w505) -> ()
                        n289 = property class="Bool (strict)"(reference=w509, "Position"=w507) -> ()  [unwired: 1 in, 2 out]
                      }
                    }
                  }
                }
              }
              frame 10 {
                # "Disco"
                # "Disco"
                # "Estado 10"
                n290 = local read "referenciaDisco"() -> (w525:refnum<vi>)
                n291 = property class="Bool (strict)"(reference=w525) -> ("Label.Text"=w526:string)  [unwired: 1 in, 2 out]
                n292 = local read "Tu numero de movimientos"() -> (w520:i16)
                n293 = Equal?(x=w526, y="1") -> (x = y?=w521:bool)
                n294 = Equal?(x=w526, y="3") -> (x = y?=w527:bool)
                n295 = Or(x=w521, y=w527) -> (x .or. y?=w522:bool)
                n296 = case shown="True" w522 {
                  tunnel: w529 -> [_ w534]
                  tunnel: [w530 w533] -> w528
                  tunnel: w521 -> [_ w532]
                  tunnel: w520 -> [_ w531]
                  frame False {
                    n297 = local read "estado"() -> (w530:u16)
                  }
                  frame True {
                    n298 = case shown="True" w532 {
                      tunnel: w534 -> [w539 w556]
                      tunnel: [w537 w554] -> w533
                      tunnel: w531 -> [w535 w552]
                      frame True {
                        # "Disco 1"
                        n299 = case shown="3" w539 {
                          tunnel: [T1 {"Left"=223, "Top"=653} ("Position") w546 T1 {"Left"=1300, "Top"=597} ("Position")] -> w538
                          tunnel: [u16 13 ("estado") w545 u16 14 ("estado")] -> w537
                          tunnel: [w543 w547 w549] -> w536
                          tunnel: w535 -> [w544 w547 w551]
                          frame 1, Default {
                            # "Torre 1"
                            n300 = Increment(x=w544) -> (x+1=w543:i16)
                          }
                          frame 2 {
                            # "Volvio a la misma\nposicion"
                            # "Torre 2"
                            n301 = local read "positionIncialDisco"() -> (w546:T1)
                            n302 = local read "estado"() -> (w545:u16)
                          }
                          frame 3 {
                            # "Torre 3"
                            n303 = Increment(x=w551) -> (x+1=w549:i16)
                          }
                        }
                        n304 = local read "referenciaDisco"() -> (w540:refnum<vi>)
                        n305 = local write "Tu numero de movimientos"(w536) -> ()
                        n306 = property class="Bool (strict)"(reference=w540, "Position"=w538) -> ()  [unwired: 1 in, 2 out]
                      }
                      frame False {
                        # "Disco 3"
                        n307 = case shown="2" w556 {
                          tunnel: [T1 {"Left"=163, "Top"=653} ("Position") w563 w566] -> w555
                          tunnel: [u16 8 ("estado") w562 w565] -> w554
                          tunnel: [w558 w564 w567] -> w553
                          tunnel: w552 -> [w561 w564 w567]
                          frame 1, Default {
                            # "Torre 1"
                            n308 = Increment(x=w561) -> (x+1=w558:i16)
                          }
                          frame 2 {
                            # "accion no valida"
                            # "Torre 2"
                            n309 = local read "positionIncialDisco"() -> (w563:T1)
                            n310 = local read "estado"() -> (w562:u16)
                          }
                          frame 3 {
                            # "Volvio a la misma\nposicion"
                            # "Torre 3"
                            n311 = local read "positionIncialDisco"() -> (w566:T1)
                            n312 = local read "estado"() -> (w565:u16)
                          }
                        }
                        n313 = local read "referenciaDisco"() -> (w557:refnum<vi>)
                        n314 = local write "Tu numero de movimientos"(w553) -> ()
                        n315 = property class="Bool (strict)"(reference=w557, "Position"=w555) -> ()  [unwired: 1 in, 2 out]
                      }
                    }
                  }
                }
              }
              frame 11 {
                # "Disco"
                # "Disco"
                # "Estado 11"
                n316 = local read "referenciaDisco"() -> (w573:refnum<vi>)
                n317 = property class="Bool (strict)"(reference=w573) -> ("Label.Text"=w574:string)  [unwired: 1 in, 2 out]
                n318 = local read "Tu numero de movimientos"() -> (w568:i16)
                n319 = Equal?(x=w574, y="1") -> (x = y?=w569:bool)
                n320 = Equal?(x=w574, y="2") -> (x = y?=w575:bool)
                n321 = Or(x=w569, y=w575) -> (x .or. y?=w570:bool)
                n322 = case shown="True" w570 {
                  tunnel: w577 -> [_ w582]
                  tunnel: [w578 w581] -> w576
                  tunnel: w569 -> [_ w580]
                  tunnel: w568 -> [_ w579]
                  frame False {
                    n323 = local read "estado"() -> (w578:u16)
                  }
                  frame True {
                    n324 = case shown="False" w580 {
                      tunnel: w582 -> [w587 w604]
                      tunnel: [w585 w602] -> w581
                      tunnel: w579 -> [w583 w600]
                      frame True {
                        # "Disco 1"
                        n325 = case shown="1, Default" w587 {
                          tunnel: [w590 T1 {"Left"=750, "Top"=597} ("Position") T1 {"Left"=1300, "Top"=597} ("Position")] -> w586
                          tunnel: [w589 u16 12 ("estado") u16 9 ("estado")] -> w585
                          tunnel: [w591 w593 w597] -> w584
                          tunnel: w583 -> [w591 w595 w599]
                          frame 1, Default {
                            # "Volvio a la misma\nposicion"
                            # "Torre 1"
                            n326 = local read "positionIncialDisco"() -> (w590:T1)
                            n327 = local read "estado"() -> (w589:u16)
                          }
                          frame 2 {
                            # "Torre 2"
                            n328 = Increment(x=w595) -> (x+1=w593:i16)
                          }
                          frame 3 {
                            # "Torre 3"
                            n329 = Increment(x=w599) -> (x+1=w597:i16)
                          }
                        }
                        n330 = local read "referenciaDisco"() -> (w588:refnum<vi>)
                        n331 = local write "Tu numero de movimientos"(w584) -> ()
                        n332 = property class="Bool (strict)"(reference=w588, "Position"=w586) -> ()  [unwired: 1 in, 2 out]
                      }
                      frame False {
                        # "Disco 2"
                        n333 = case shown="2" w604 {
                          tunnel: [w607 T1 {"Left"=718, "Top"=597} ("positionIncialDisco") w614] -> w603
                          tunnel: [w606 u16 15 ("estado") w613] -> w602
                          tunnel: [w608 w611 w615] -> w601
                          tunnel: w600 -> [w608 w612 w615]
                          frame 1, Default {
                            # "accion no valida"
                            # "Torre 1"
                            n334 = local read "positionIncialDisco"() -> (w607:T1)
                            n335 = local read "estado"() -> (w606:u16)
                          }
                          frame 2 {
                            # "Torre 2"
                            n336 = Increment(x=w612) -> (x+1=w611:i16)
                          }
                          frame 3 {
                            # "Volvio a la misma\nposicion"
                            # "Torre 3"
                            n337 = local read "positionIncialDisco"() -> (w614:T1)
                            n338 = local read "estado"() -> (w613:u16)
                          }
                        }
                        n339 = local read "referenciaDisco"() -> (w605:refnum<vi>)
                        n340 = local write "Tu numero de movimientos"(w601) -> ()
                        n341 = property class="Bool (strict)"(reference=w605, "Position"=w603) -> ()  [unwired: 1 in, 2 out]
                      }
                    }
                  }
                }
              }
              frame 12 {
                # "Disco"
                # "Disco"
                # "Estado 12"
                n342 = local read "referenciaDisco"() -> (w621:refnum<vi>)
                n343 = property class="Bool (strict)"(reference=w621) -> ("Label.Text"=w622:string)  [unwired: 1 in, 2 out]
                n344 = local read "Tu numero de movimientos"() -> (w616:i16)
                n345 = Equal?(x=w622, y="1") -> (x = y?=w617:bool)
                n346 = Equal?(x=w622, y="2") -> (x = y?=w623:bool)
                n347 = Or(x=w617, y=w623) -> (x .or. y?=w618:bool)
                n348 = case shown="True" w618 {
                  tunnel: w625 -> [_ w630]
                  tunnel: [w626 w629] -> w624
                  tunnel: w617 -> [_ w628]
                  tunnel: w616 -> [_ w627]
                  frame False {
                    n349 = local read "estado"() -> (w626:u16)
                  }
                  frame True {
                    n350 = case shown="False" w628 {
                      tunnel: w630 -> [w635 w652]
                      tunnel: [w633 w650] -> w629
                      tunnel: w627 -> [w631 w648]
                      frame True {
                        # "Disco 1"
                        n351 = case shown="3" w635 {
                          tunnel: [T1 {"Left"=223, "Top"=653} ("Position") w642 T1 {"Left"=1300, "Top"=597} ("Position")] -> w634
                          tunnel: [u16 11 ("estado") w641 u16 9 ("estado")] -> w633
                          tunnel: [w638 w643 w645] -> w632
                          tunnel: w631 -> [w640 w643 w647]
                          frame 1, Default {
                            # "Torre 1"
                            n352 = Increment(x=w640) -> (x+1=w638:i16)
                          }
                          frame 2 {
                            # "Volvio a la misma\nposicion"
                            # "Torre 2"
                            n353 = local read "positionIncialDisco"() -> (w642:T1)
                            n354 = local read "estado"() -> (w641:u16)
                          }
                          frame 3 {
                            # "Torre 3"
                            n355 = Increment(x=w647) -> (x+1=w645:i16)
                          }
                        }
                        n356 = local read "referenciaDisco"() -> (w636:refnum<vi>)
                        n357 = local write "Tu numero de movimientos"(w632) -> ()
                        n358 = property class="Bool (strict)"(reference=w636, "Position"=w634) -> ()  [unwired: 1 in, 2 out]
                      }
                      frame False {
                        # "Disco 2"
                        n359 = case shown="1, Default" w652 {
                          tunnel: [T1 {"Left"=193, "Top"=653} ("Position") w659 w662] -> w651
                          tunnel: [u16 16 ("estado") w658 w661] -> w650
                          tunnel: [w656 w660 w663] -> w649
                          tunnel: w648 -> [w657 w660 w663]
                          frame 1, Default {
                            # "Torre 1"
                            n360 = Increment(x=w657) -> (x+1=w656:i16)
                          }
                          frame 2 {
                            # "accion no valida"
                            # "Torre 2"
                            n361 = local read "positionIncialDisco"() -> (w659:T1)
                            n362 = local read "estado"() -> (w658:u16)
                          }
                          frame 3 {
                            # "Volvio a la misma\nposicion"
                            # "Torre 3"
                            n363 = local read "positionIncialDisco"() -> (w662:T1)
                            n364 = local read "estado"() -> (w661:u16)
                          }
                        }
                        n365 = local read "referenciaDisco"() -> (w653:refnum<vi>)
                        n366 = local write "Tu numero de movimientos"(w649) -> ()
                        n367 = property class="Bool (strict)"(reference=w653, "Position"=w651) -> ()  [unwired: 1 in, 2 out]
                      }
                    }
                  }
                }
              }
              frame 13 {
                # "Disco"
                # "Disco"
                # "Estado 13"
                n368 = local read "referenciaDisco"() -> (w669:refnum<vi>)
                n369 = property class="Bool (strict)"(reference=w669) -> ("Label.Text"=w670:string)  [unwired: 1 in, 2 out]
                n370 = local read "Tu numero de movimientos"() -> (w664:i16)
                n371 = Equal?(x=w670, y="1") -> (x = y?=w665:bool)
                n372 = Equal?(x=w670, y="2") -> (x = y?=w671:bool)
                n373 = Or(x=w665, y=w671) -> (x .or. y?=w666:bool)
                n374 = case shown="True" w666 {
                  tunnel: w673 -> [_ w678]
                  tunnel: [w674 w677] -> w672
                  tunnel: w665 -> [_ w676]
                  tunnel: w664 -> [_ w675]
                  frame False {
                    n375 = local read "estado"() -> (w674:u16)
                  }
                  frame True {
                    n376 = case shown="False" w676 {
                      tunnel: w678 -> [w683 w700]
                      tunnel: [w681 w698] -> w677
                      tunnel: w675 -> [w679 w696]
                      frame True {
                        # "Disco 1"
                        n377 = case shown="3" w683 {
                          tunnel: [w686 T1 {"Left"=750, "Top"=597} ("Position") T1 {"Left"=1300, "Top"=597} ("Position")] -> w682
                          tunnel: [w685 u16 10 ("estado") u16 14 ("estado")] -> w681
                          tunnel: [w687 w690 w693] -> w680
                          tunnel: w679 -> [w687 w691 w695]
                          frame 1, Default {
                            # "Volvio a la misma\nposicion"
                            # "Torre 1"
                            n378 = local read "positionIncialDisco"() -> (w686:T1)
                            n379 = local read "estado"() -> (w685:u16)
                          }
                          frame 2 {
                            # "Torre 2"
                            n380 = Increment(x=w691) -> (x+1=w690:i16)
                          }
                          frame 3 {
                            # "Torre 3"
                            n381 = Increment(x=w695) -> (x+1=w693:i16)
                          }
                        }
                        n382 = local read "referenciaDisco"() -> (w684:refnum<vi>)
                        n383 = local write "Tu numero de movimientos"(w680) -> ()
                        n384 = property class="Bool (strict)"(reference=w684, "Position"=w682) -> ()  [unwired: 1 in, 2 out]
                      }
                      frame False {
                        # "Disco 2"
                        n385 = case shown="3" w700 {
                          tunnel: [w703 w706 T1 {"Left"=1270, "Top"=597} ("Position")] -> w699
                          tunnel: [w702 w705 u16 18 ("estado")] -> w698
                          tunnel: [w704 w707 w710] -> w697
                          tunnel: w696 -> [w704 w707 w711]
                          frame 1, Default {
                            # "accion no valida"
                            # "Torre 1"
                            n386 = local read "positionIncialDisco"() -> (w703:T1)
                            n387 = local read "estado"() -> (w702:u16)
                          }
                          frame 2 {
                            # "Volvio a la misma\nposicion"
                            # "Torre 2"
                            n388 = local read "positionIncialDisco"() -> (w706:T1)
                            n389 = local read "estado"() -> (w705:u16)
                          }
                          frame 3 {
                            # "Torre 3"
                            n390 = Increment(x=w711) -> (x+1=w710:i16)
                          }
                        }
                        n391 = local read "referenciaDisco"() -> (w701:refnum<vi>)
                        n392 = local write "Tu numero de movimientos"(w697) -> ()
                        n393 = property class="Bool (strict)"(reference=w701, "Position"=w699) -> ()  [unwired: 1 in, 2 out]
                      }
                    }
                  }
                }
              }
              frame 14 {
                # "Disco"
                # "Disco"
                # "Estado 14"
                n394 = local read "referenciaDisco"() -> (w717:refnum<vi>)
                n395 = property class="Bool (strict)"(reference=w717) -> ("Label.Text"=w718:string)  [unwired: 1 in, 2 out]
                n396 = local read "Tu numero de movimientos"() -> (w712:i16)
                n397 = Equal?(x=w718, y="1") -> (x = y?=w713:bool)
                n398 = Equal?(x=w718, y="2") -> (x = y?=w719:bool)
                n399 = Or(x=w713, y=w719) -> (x .or. y?=w714:bool)
                n400 = case shown="True" w714 {
                  tunnel: w721 -> [_ w726]
                  tunnel: [w722 w725] -> w720
                  tunnel: w713 -> [_ w724]
                  tunnel: w712 -> [_ w723]
                  frame False {
                    n401 = local read "estado"() -> (w722:u16)
                  }
                  frame True {
                    n402 = case shown="False" w724 {
                      tunnel: w726 -> [w731 w748]
                      tunnel: [w729 w746] -> w725
                      tunnel: w723 -> [w727 w744]
                      frame True {
                        # "Disco 1"
                        n403 = case shown="3" w731 {
                          tunnel: [T1 {"Left"=223, "Top"=653} ("Position") T1 {"Left"=750, "Top"=597} ("Position") w742] -> w730
                          tunnel: [u16 13 ("estado") u16 10 ("estado") w741] -> w729
                          tunnel: [w735 w739 w743] -> w728
                          tunnel: w727 -> [w736 w740 w743]
                          frame 1, Default {
                            # "Torre 1"
                            n404 = Increment(x=w736) -> (x+1=w735:i16)
                          }
                          frame 2 {
                            # "Torre 2"
                            n405 = Increment(x=w740) -> (x+1=w739:i16)
                          }
                          frame 3 {
                            # "Volvio a la misma\nposicion"
                            # "Torre 3"
                            n406 = local read "positionIncialDisco"() -> (w742:T1)
                            n407 = local read "estado"() -> (w741:u16)
                          }
                        }
                        n408 = local read "referenciaDisco"() -> (w732:refnum<vi>)
                        n409 = local write "Tu numero de movimientos"(w728) -> ()
                        n410 = property class="Bool (strict)"(reference=w732, "Position"=w730) -> ()  [unwired: 1 in, 2 out]
                      }
                      frame False {
                        # "Disco 2"
                        n411 = case shown="1, Default" w748 {
                          tunnel: [T1 {"Left"=193, "Top"=653} ("Position") w755 w758] -> w747
                          tunnel: [u16 19 ("estado") w754 w757] -> w746
                          tunnel: [w752 w756 w759] -> w745
                          tunnel: w744 -> [w753 w756 w759]
                          frame 1, Default {
                            # "Torre 1"
                            n412 = Increment(x=w753) -> (x+1=w752:i16)
                          }
                          frame 2 {
                            # "Volvio a la misma\nposicion"
                            # "Torre 2"
                            n413 = local read "positionIncialDisco"() -> (w755:T1)
                            n414 = local read "estado"() -> (w754:u16)
                          }
                          frame 3 {
                            # "accion no valida"
                            # "Torre 3"
                            n415 = local read "positionIncialDisco"() -> (w758:T1)
                            n416 = local read "estado"() -> (w757:u16)
                          }
                        }
                        n417 = local read "referenciaDisco"() -> (w749:refnum<vi>)
                        n418 = local write "Tu numero de movimientos"(w745) -> ()
                        n419 = property class="Bool (strict)"(reference=w749, "Position"=w747) -> ()  [unwired: 1 in, 2 out]
                      }
                    }
                  }
                }
              }
              frame 15 {
                # "Disco"
                # "Disco"
                # "Estado 15"
                n420 = local read "referenciaDisco"() -> (w765:refnum<vi>)
                n421 = property class="Bool (strict)"(reference=w765) -> ("Label.Text"=w766:string)  [unwired: 1 in, 2 out]
                n422 = local read "Tu numero de movimientos"() -> (w760:i16)
                n423 = Equal?(x=w766, y="1") -> (x = y?=w761:bool)
                n424 = Equal?(x=w766, y="2") -> (x = y?=w767:bool)
                n425 = Or(x=w761, y=w767) -> (x .or. y?=w762:bool)
                n426 = case shown="True" w762 {
                  tunnel: w769 -> [_ w774]
                  tunnel: [w770 w773] -> w768
                  tunnel: w761 -> [_ w772]
                  tunnel: w760 -> [_ w771]
                  frame False {
                    n427 = local read "estado"() -> (w770:u16)
                  }
                  frame True {
                    n428 = case shown="True" w772 {
                      tunnel: w774 -> [w779 w796]
                      tunnel: [w777 w794] -> w773
                      tunnel: w771 -> [w775 w792]
                      frame True {
                        # "Disco 1"
                        n429 = case shown="3" w779 {
                          tunnel: [w782 T1 {"Left"=750, "Top"=541} ("Position") T1 {"Left"=1300, "Top"=653} ("Position")] -> w778
                          tunnel: [w781 u16 20 ("estado") u16 21 ("estado")] -> w777
                          tunnel: [w783 w786 w789] -> w776
                          tunnel: w775 -> [w783 w787 w791]
                          frame 1, Default {
                            # "Volvio a la misma\nposicion"
                            # "Torre 1"
                            n430 = local read "positionIncialDisco"() -> (w782:T1)
                            n431 = local read "estado"() -> (w781:u16)
                          }
                          frame 2 {
                            # "Torre 2"
                            n432 = Increment(x=w787) -> (x+1=w786:i16)
                          }
                          frame 3 {
                            # "Torre 3"
                            n433 = Increment(x=w791) -> (x+1=w789:i16)
                          }
                        }
                        n434 = local read "referenciaDisco"() -> (w780:refnum<vi>)
                        n435 = local write "Tu numero de movimientos"(w776) -> ()
                        n436 = property class="Bool (strict)"(reference=w780, "Position"=w778) -> ()  [unwired: 1 in, 2 out]
                      }
                      frame False {
                        # "Disco 2"
                        n437 = case shown="3" w796 {
                          tunnel: [w799 w802 T1 {"Left"=1270, "Top"=653} ("Position")] -> w795
                          tunnel: [w798 w801 u16 11 ("estado")] -> w794
                          tunnel: [w800 w803 w805] -> w793
                          tunnel: w792 -> [w800 w803 w807]
                          frame 1, Default {
                            # "accion no valida"
                            # "Torre 1"
                            n438 = local read "positionIncialDisco"() -> (w799:T1)
                            n439 = local read "estado"() -> (w798:u16)
                          }
                          frame 2 {
                            # "Volvio a la misma\nposicion"
                            # "Torre 2"
                            n440 = local read "positionIncialDisco"() -> (w802:T1)
                            n441 = local read "estado"() -> (w801:u16)
                          }
                          frame 3 {
                            # "Torre 3"
                            n442 = Increment(x=w807) -> (x+1=w805:i16)
                          }
                        }
                        n443 = local read "referenciaDisco"() -> (w797:refnum<vi>)
                        n444 = local write "Tu numero de movimientos"(w793) -> ()
                        n445 = property class="Bool (strict)"(reference=w797, "Position"=w795) -> ()  [unwired: 1 in, 2 out]
                      }
                    }
                  }
                }
              }
              frame 16 {
                # "Disco"
                # "Disco"
                # "Estado 16"
                n446 = local read "referenciaDisco"() -> (w813:refnum<vi>)
                n447 = property class="Bool (strict)"(reference=w813) -> ("Label.Text"=w814:string)  [unwired: 1 in, 2 out]
                n448 = local read "Tu numero de movimientos"() -> (w808:i16)
                n449 = Equal?(x=w814, y="1") -> (x = y?=w809:bool)
                n450 = Equal?(x=w814, y="2") -> (x = y?=w815:bool)
                n451 = Or(x=w809, y=w815) -> (x .or. y?=w810:bool)
                n452 = case shown="True" w810 {
                  tunnel: w817 -> [_ w822]
                  tunnel: [w818 w821] -> w816
                  tunnel: w809 -> [_ w820]
                  tunnel: w808 -> [_ w819]
                  frame False {
                    n453 = local read "estado"() -> (w818:u16)
                  }
                  frame True {
                    n454 = case shown="True" w820 {
                      tunnel: w822 -> [w827 w844]
                      tunnel: [w825 w842] -> w821
                      tunnel: w819 -> [w823 w840]
                      frame True {
                        # "Disco 1"
                        n455 = case shown="1, Default" w827 {
                          tunnel: [T1 {"Left"=223, "Top"=597} ("Position") w834 T1 {"Left"=1300, "Top"=653} ("Position")] -> w826
                          tunnel: [u16 22 ("estado") w833 u16 23 ("estado")] -> w825
                          tunnel: [w830 w835 w837] -> w824
                          tunnel: w823 -> [w832 w835 w839]
                          frame 1, Default {
                            # "Torre 1"
                            n456 = Increment(x=w832) -> (x+1=w830:i16)
                          }
                          frame 2 {
                            # "Volvio a la misma\nposicion"
                            # "Torre 2"
                            n457 = local read "positionIncialDisco"() -> (w834:T1)
                            n458 = local read "estado"() -> (w833:u16)
                          }
                          frame 3 {
                            # "Torre 3"
                            n459 = Increment(x=w839) -> (x+1=w837:i16)
                          }
                        }
                        n460 = local read "referenciaDisco"() -> (w828:refnum<vi>)
                        n461 = local write "Tu numero de movimientos"(w824) -> ()
                        n462 = property class="Bool (strict)"(reference=w828, "Position"=w826) -> ()  [unwired: 1 in, 2 out]
                      }
                      frame False {
                        # "Disco 2"
                        n463 = case shown="3" w844 {
                          tunnel: [w847 w850 T1 {"Left"=1270, "Top"=653} ("Position")] -> w843
                          tunnel: [w846 w849 u16 12 ("estado")] -> w842
                          tunnel: [w848 w851 w853] -> w841
                          tunnel: w840 -> [w848 w851 w855]
                          frame 1, Default {
                            # "Volvio a la misma\nposicion"
                            # "Torre 1"
                            n464 = local read "positionIncialDisco"() -> (w847:T1)
                            n465 = local read "estado"() -> (w846:u16)
                          }
                          frame 2 {
                            # "accion no valida"
                            # "Torre 2"
                            n466 = local read "positionIncialDisco"() -> (w850:T1)
                            n467 = local read "estado"() -> (w849:u16)
                          }
                          frame 3 {
                            # "Torre 3"
                            n468 = Increment(x=w855) -> (x+1=w853:i16)
                          }
                        }
                        n469 = local read "referenciaDisco"() -> (w845:refnum<vi>)
                        n470 = local write "Tu numero de movimientos"(w841) -> ()
                        n471 = property class="Bool (strict)"(reference=w845, "Position"=w843) -> ()  [unwired: 1 in, 2 out]
                      }
                    }
                  }
                }
              }
              frame 17 {
                # "Disco"
                # "Disco"
                # "Estado 17\nes igual al Estado 10"
                n472 = local read "referenciaDisco"() -> (w861:refnum<vi>)
                n473 = property class="Bool (strict)"(reference=w861) -> ("Label.Text"=w862:string)  [unwired: 1 in, 2 out]
                n474 = local read "Tu numero de movimientos"() -> (w856:i16)
                n475 = Equal?(x=w862, y="1") -> (x = y?=w857:bool)
                n476 = Equal?(x=w862, y="3") -> (x = y?=w863:bool)
                n477 = Or(x=w857, y=w863) -> (x .or. y?=w858:bool)
                n478 = case shown="True" w858 {
                  tunnel: w865 -> [_ w870]
                  tunnel: [w866 w869] -> w864
                  tunnel: w857 -> [_ w868]
                  tunnel: w856 -> [_ w867]
                  frame False {
                    n479 = local read "estado"() -> (w866:u16)
                  }
                  frame True {
                    n480 = case shown="True" w868 {
                      tunnel: w870 -> [w875 w892]
                      tunnel: [w873 w890] -> w869
                      tunnel: w867 -> [w871 w888]
                      frame True {
                        # "Disco 1"
                        n481 = case shown="1, Default" w875 {
                          tunnel: [T1 {"Left"=223, "Top"=653} ("Position") w882 T1 {"Left"=1300, "Top"=597} ("Position")] -> w874
                          tunnel: [u16 13 ("estado") w881 u16 14 ("estado")] -> w873
                          tunnel: [w879 w883 w885] -> w872
                          tunnel: w871 -> [w880 w883 w887]
                          frame 1, Default {
                            # "Torre 1"
                            n482 = Increment(x=w880) -> (x+1=w879:i16)
                          }
                          frame 2 {
                            # "Volvio a la misma\nposicion"
                            # "Torre 2"
                            n483 = local read "positionIncialDisco"() -> (w882:T1)
                            n484 = local read "estado"() -> (w881:u16)
                          }
                          frame 3 {
                            # "Torre 3"
                            n485 = Increment(x=w887) -> (x+1=w885:i16)
                          }
                        }
                        n486 = local read "referenciaDisco"() -> (w876:refnum<vi>)
                        n487 = local write "Tu numero de movimientos"(w872) -> ()
                        n488 = property class="Bool (strict)"(reference=w876, "Position"=w874) -> ()  [unwired: 1 in, 2 out]
                      }
                      frame False {
                        # "Disco 3"
                        n489 = case shown="2" w892 {
                          tunnel: [T1 {"Left"=163, "Top"=653} ("Position") w899 w902] -> w891
                          tunnel: [u16 8 ("estado") w898 w901] -> w890
                          tunnel: [w894 w900 w903] -> w889
                          tunnel: w888 -> [w897 w900 w903]
                          frame 1, Default {
                            # "Torre 1"
                            n490 = Increment(x=w897) -> (x+1=w894:i16)
                          }
                          frame 2 {
                            # "accion no valida"
                            # "Torre 2"
                            n491 = local read "positionIncialDisco"() -> (w899:T1)
                            n492 = local read "estado"() -> (w898:u16)
                          }
                          frame 3 {
                            # "Volvio a la misma\nposicion"
                            # "Torre 3"
                            n493 = local read "positionIncialDisco"() -> (w902:T1)
                            n494 = local read "estado"() -> (w901:u16)
                          }
                        }
                        n495 = local read "referenciaDisco"() -> (w893:refnum<vi>)
                        n496 = local write "Tu numero de movimientos"(w889) -> ()
                        n497 = property class="Bool (strict)"(reference=w893, "Position"=w891) -> ()  [unwired: 1 in, 2 out]
                      }
                    }
                  }
                }
              }
              frame 18 {
                # "Disco"
                # "Disco"
                # "Estado 18"
                n498 = local read "referenciaDisco"() -> (w909:refnum<vi>)
                n499 = property class="Bool (strict)"(reference=w909) -> ("Label.Text"=w910:string)  [unwired: 1 in, 2 out]
                n500 = local read "Tu numero de movimientos"() -> (w904:i16)
                n501 = Equal?(x=w910, y="1") -> (x = y?=w905:bool)
                n502 = Equal?(x=w910, y="2") -> (x = y?=w911:bool)
                n503 = Or(x=w905, y=w911) -> (x .or. y?=w906:bool)
                n504 = case shown="True" w906 {
                  tunnel: w913 -> [_ w918]
                  tunnel: [w914 w917] -> w912
                  tunnel: w905 -> [_ w916]
                  tunnel: w904 -> [_ w915]
                  frame False {
                    n505 = local read "estado"() -> (w914:u16)
                  }
                  frame True {
                    n506 = case shown="True" w916 {
                      tunnel: w918 -> [w923 w940]
                      tunnel: [w921 w938] -> w917
                      tunnel: w915 -> [w919 w936]
                      frame True {
                        # "Disco 1"
                        n507 = case shown="2" w923 {
                          tunnel: [w926 T1 {"Left"=750, "Top"=653} ("Position") T1 {"Left"=1300, "Top"=541} ("Position")] -> w922
                          tunnel: [w925 u16 24 ("estado") u16 25 ("estado")] -> w921
                          tunnel: [w927 w929 w933] -> w920
                          tunnel: w919 -> [w927 w931 w935]
                          frame 1, Default {
                            # "Volvio a la misma\nposicion"
                            # "Torre 1"
                            n508 = local read "positionIncialDisco"() -> (w926:T1)
                            n509 = local read "estado"() -> (w925:u16)
                          }
                          frame 2 {
                            # "Torre 2"
                            n510 = Increment(x=w931) -> (x+1=w929:i16)
                          }
                          frame 3 {
                            # "Torre 3"
                            n511 = Increment(x=w935) -> (x+1=w933:i16)
                          }
                        }
                        n512 = local read "referenciaDisco"() -> (w924:refnum<vi>)
                        n513 = local write "Tu numero de movimientos"(w920) -> ()
                        n514 = property class="Bool (strict)"(reference=w924, "Position"=w922) -> ()  [unwired: 1 in, 2 out]
                      }
                      frame False {
                        # "Disco 2"
                        n515 = case shown="2" w940 {
                          tunnel: [w943 T1 {"Left"=720, "Top"=653} ("Position") w949] -> w939
                          tunnel: [w942 u16 13 ("estado") w950] -> w938
                          tunnel: [w944 w946 w951] -> w937
                          tunnel: w936 -> [w944 w948 w951]
                          frame 1, Default {
                            # "accion no valida"
                            # "Torre 1"
                            n516 = local read "positionIncialDisco"() -> (w943:T1)
                            n517 = local read "estado"() -> (w942:u16)
                          }
                          frame 2 {
                            # "Torre 2"
                            n518 = Increment(x=w948) -> (x+1=w946:i16)
                          }
                          frame 3 {
                            # "accion no valida"
                            # "Torre 3"
                            n519 = local read "positionIncialDisco"() -> (w949:T1)
                            n520 = local read "estado"() -> (w950:u16)
                          }
                        }
                        n521 = local read "referenciaDisco"() -> (w941:refnum<vi>)
                        n522 = local write "Tu numero de movimientos"(w937) -> ()
                        n523 = property class="Bool (strict)"(reference=w941, "Position"=w939) -> ()  [unwired: 1 in, 2 out]
                      }
                    }
                  }
                }
              }
              frame 19 {
                # "Disco"
                # "Disco"
                # "Estado 19"
                n524 = local read "referenciaDisco"() -> (w957:refnum<vi>)
                n525 = property class="Bool (strict)"(reference=w957) -> ("Label.Text"=w958:string)  [unwired: 1 in, 2 out]
                n526 = local read "Tu numero de movimientos"() -> (w952:i16)
                n527 = Equal?(x=w958, y="1") -> (x = y?=w953:bool)
                n528 = Equal?(x=w958, y="2") -> (x = y?=w959:bool)
                n529 = Or(x=w953, y=w959) -> (x .or. y?=w954:bool)
                n530 = case shown="True" w954 {
                  tunnel: w961 -> [_ w966]
                  tunnel: [w962 w965] -> w960
                  tunnel: w953 -> [_ w964]
                  tunnel: w952 -> [_ w963]
                  frame False {
                    n531 = local read "estado"() -> (w962:u16)
                  }
                  frame True {
                    n532 = case shown="True" w964 {
                      tunnel: w966 -> [w971 w988]
                      tunnel: [w969 w986] -> w965
                      tunnel: w963 -> [w967 w984]
                      frame True {
                        # "Disco 1"
                        n533 = case shown="1, Default" w971 {
                          tunnel: [T1 {"Left"=223, "Top"=597} ("Position") T1 {"Left"=750, "Top"=653} ("Position") w982] -> w970
                          tunnel: [u16 26 ("estado") u16 27 ("estado") w981] -> w969
                          tunnel: [w975 w979 w983] -> w968
                          tunnel: w967 -> [w976 w980 w983]
                          frame 1, Default {
                            # "Torre 1"
                            n534 = Increment(x=w976) -> (x+1=w975:i16)
                          }
                          frame 2 {
                            # "Torre 2"
                            n535 = Increment(x=w980) -> (x+1=w979:i16)
                          }
                          frame 3 {
                            # "Volvio a la misma\nposicion"
                            # "Torre 3"
                            n536 = local read "positionIncialDisco"() -> (w982:T1)
                            n537 = local read "estado"() -> (w981:u16)
                          }
                        }
                        n538 = local read "referenciaDisco"() -> (w972:refnum<vi>)
                        n539 = local write "Tu numero de movimientos"(w968) -> ()
                        n540 = property class="Bool (strict)"(reference=w972, "Position"=w970) -> ()  [unwired: 1 in, 2 out]
                      }
                      frame False {
                        # "Disco 2"
                        n541 = case shown="3" w988 {
                          tunnel: [w991 T1 {"Left"=720, "Top"=653} ("Position") w997] -> w987
                          tunnel: [w990 u16 14 ("estado") w998] -> w986
                          tunnel: [w992 w994 w999] -> w985
                          tunnel: w984 -> [w992 w996 w999]
                          frame 1, Default {
                            # "Volvio a la misma\nposicion"
                            # "Torre 1"
                            n542 = local read "positionIncialDisco"() -> (w991:T1)
                            n543 = local read "estado"() -> (w990:u16)
                          }
                          frame 2 {
                            # "Torre 2"
                            n544 = Increment(x=w996) -> (x+1=w994:i16)
                          }
                          frame 3 {
                            # "accion no valida"
                            # "Torre 3"
                            n545 = local read "positionIncialDisco"() -> (w997:T1)
                            n546 = local read "estado"() -> (w998:u16)
                          }
                        }
                        n547 = local read "referenciaDisco"() -> (w989:refnum<vi>)
                        n548 = local write "Tu numero de movimientos"(w985) -> ()
                        n549 = property class="Bool (strict)"(reference=w989, "Position"=w987) -> ()  [unwired: 1 in, 2 out]
                      }
                    }
                  }
                }
              }
              frame 20 {
                # "Disco"
                # "Disco"
                # "Estado 20"
                n550 = local read "referenciaDisco"() -> (w1005:refnum<vi>)
                n551 = property class="Bool (strict)"(reference=w1005) -> ("Label.Text"=w1006:string)  [unwired: 1 in, 2 out]
                n552 = local read "Tu numero de movimientos"() -> (w1000:i16)
                n553 = Equal?(x=w1006, y="1") -> (x = y?=w1001:bool)
                n554 = Equal?(x=w1006, y="1") -> (x = y?=w1007:bool)
                n555 = Or(x=w1001, y=w1007) -> (x .or. y?=w1002:bool)
                n556 = case shown="True" w1002 {
                  tunnel: w1009 -> [_ w1016]
                  tunnel: [w1010 w1015] -> w1008
                  tunnel: w1000 -> [_ w1014]
                  frame False {
                    n557 = local read "estado"() -> (w1010:u16)
                  }
                  frame True {
                    # "Disco 1"
                    n558 = case shown="1, Default" w1016 {
                      tunnel: [T1 {"Left"=223, "Top"=653} ("Position") w1022 T1 {"Left"=1300, "Top"=653} ("Position")] -> w1012
                      tunnel: [u16 15 ("estado") w1021 u16 21 ("estado")] -> w1015
                      tunnel: [w1019 w1023 w1026] -> w1011
                      tunnel: w1014 -> [w1020 w1023 w1027]
                      frame 1, Default {
                        # "Torre 1"
                        n559 = Increment(x=w1020) -> (x+1=w1019:i16)
                      }
                      frame 2 {
                        # "Volvio a la misma\nposicion"
                        # "Torre 2"
                        n560 = local read "positionIncialDisco"() -> (w1022:T1)
                        n561 = local read "estado"() -> (w1021:u16)
                      }
                      frame 3 {
                        # "Torre 3"
                        n562 = Increment(x=w1027) -> (x+1=w1026:i16)
                      }
                    }
                    n563 = local read "referenciaDisco"() -> (w1013:refnum<vi>)
                    n564 = local write "Tu numero de movimientos"(w1011) -> ()
                    n565 = property class="Bool (strict)"(reference=w1013, "Position"=w1012) -> ()  [unwired: 1 in, 2 out]
                  }
                }
              }
              frame 21 {
                # "Disco"
                # "Disco"
                # "Estado 21"
                n566 = local read "referenciaDisco"() -> (w1033:refnum<vi>)
                n567 = property class="Bool (strict)"(reference=w1033) -> ("Label.Text"=w1034:string)  [unwired: 1 in, 2 out]
                n568 = local read "Tu numero de movimientos"() -> (w1028:i16)
                n569 = Equal?(x=w1034, y="1") -> (x = y?=w1029:bool)
                n570 = Equal?(x=w1034, y="2") -> (x = y?=w1035:bool)
                n571 = Or(x=w1029, y=w1035) -> (x .or. y?=w1030:bool)
                n572 = case shown="True" w1030 {
                  tunnel: w1037 -> [_ w1042]
                  tunnel: [w1038 w1041] -> w1036
                  tunnel: w1029 -> [_ w1040]
                  tunnel: w1028 -> [_ w1039]
                  frame False {
                    n573 = local read "estado"() -> (w1038:u16)
                  }
                  frame True {
                    n574 = case shown="False" w1040 {
                      tunnel: w1042 -> [w1047 w1064]
                      tunnel: [w1045 w1062] -> w1041
                      tunnel: w1039 -> [w1043 w1060]
                      frame True {
                        # "Disco 1"
                        n575 = case shown="3" w1047 {
                          tunnel: [T1 {"Left"=223, "Top"=653} ("Position") T1 {"Left"=750, "Top"=541} ("Position") w1058] -> w1046
                          tunnel: [u16 15 ("estado") u16 20 ("estado") w1057] -> w1045
                          tunnel: [w1051 w1055 w1059] -> w1044
                          tunnel: w1043 -> [w1052 w1056 w1059]
                          frame 1, Default {
                            # "Torre 1"
                            n576 = Increment(x=w1052) -> (x+1=w1051:i16)
                          }
                          frame 2 {
                            # "Torre 2"
                            n577 = Increment(x=w1056) -> (x+1=w1055:i16)
                          }
                          frame 3 {
                            # "Volvio a la misma\nposicion"
                            # "Torre 3"
                            n578 = local read "positionIncialDisco"() -> (w1058:T1)
                            n579 = local read "estado"() -> (w1057:u16)
                          }
                        }
                        n580 = local read "referenciaDisco"() -> (w1048:refnum<vi>)
                        n581 = local write "Tu numero de movimientos"(w1044) -> ()
                        n582 = property class="Bool (strict)"(reference=w1048, "Position"=w1046) -> ()  [unwired: 1 in, 2 out]
                      }
                      frame False {
                        # "Disco 2"
                        n583 = case shown="1, Default" w1064 {
                          tunnel: [T1 {"Left"=193, "Top"=653} ("Position") w1071 w1073] -> w1063
                          tunnel: [u16 23 ("estado") w1070 w1074] -> w1062
                          tunnel: [w1068 w1072 w1075] -> w1061
                          tunnel: w1060 -> [w1069 w1072 w1075]
                          frame 1, Default {
                            # "Torre 1"
                            n584 = Increment(x=w1069) -> (x+1=w1068:i16)
                          }
                          frame 2 {
                            # "Volvio a la misma\nposicion"
                            # "Torre 2"
                            n585 = local read "positionIncialDisco"() -> (w1071:T1)
                            n586 = local read "estado"() -> (w1070:u16)
                          }
                          frame 3 {
                            # "accion no valida"
                            # "Torre 3"
                            n587 = local read "positionIncialDisco"() -> (w1073:T1)
                            n588 = local read "estado"() -> (w1074:u16)
                          }
                        }
                        n589 = local read "referenciaDisco"() -> (w1065:refnum<vi>)
                        n590 = local write "Tu numero de movimientos"(w1061) -> ()
                        n591 = property class="Bool (strict)"(reference=w1065, "Position"=w1063) -> ()  [unwired: 1 in, 2 out]
                      }
                    }
                  }
                }
              }
              frame 22 {
                # "Disco"
                # "Disco"
                # "Estado 22"
                n592 = local read "referenciaDisco"() -> (w1081:refnum<vi>)
                n593 = property class="Bool (strict)"(reference=w1081) -> ("Label.Text"=w1082:string)  [unwired: 1 in, 2 out]
                n594 = local read "Tu numero de movimientos"() -> (w1076:i16)
                n595 = Equal?(x=w1082, y="1") -> (x = y?=w1077:bool)
                n596 = Equal?(x=w1082, y="3") -> (x = y?=w1083:bool)
                n597 = Or(x=w1077, y=w1083) -> (x .or. y?=w1078:bool)
                n598 = case shown="True" w1078 {
                  tunnel: w1085 -> [_ w1090]
                  tunnel: [w1086 w1089] -> w1084
                  tunnel: w1077 -> [_ w1088]
                  tunnel: w1076 -> [_ w1087]
                  frame False {
                    n599 = local read "estado"() -> (w1086:u16)
                  }
                  frame True {
                    n600 = case shown="False" w1088 {
                      tunnel: w1090 -> [w1095 w1112]
                      tunnel: [w1093 w1110] -> w1089
                      tunnel: w1087 -> [w1091 w1108]
                      frame True {
                        # "Disco 1"
                        n601 = case shown="3" w1095 {
                          tunnel: [w1098 T1 {"Left"=750, "Top"=597} ("Position") T1 {"Left"=1300, "Top"=653} ("Position")] -> w1094
                          tunnel: [w1097 u16 16 ("estado") u16 23 ("estado")] -> w1093
                          tunnel: [w1099 w1102 w1106] -> w1092
                          tunnel: w1091 -> [w1099 w1103 w1107]
                          frame 1, Default {
                            # "Volvio a la misma\nposicion"
                            # "Torre 1"
                            n602 = local read "positionIncialDisco"() -> (w1098:T1)
                            n603 = local read "estado"() -> (w1097:u16)
                          }
                          frame 2 {
                            # "Torre 2"
                            n604 = Increment(x=w1103) -> (x+1=w1102:i16)
                          }
                          frame 3 {
                            # "Torre 3"
                            n605 = Increment(x=w1107) -> (x+1=w1106:i16)
                          }
                        }
                        n606 = local read "referenciaDisco"() -> (w1096:refnum<vi>)
                        n607 = local write "Tu numero de movimientos"(w1092) -> ()
                        n608 = property class="Bool (strict)"(reference=w1096, "Position"=w1094) -> ()  [unwired: 1 in, 2 out]
                      }
                      frame False {
                        # "Disco 3"
                        n609 = case shown="3" w1112 {
                          tunnel: [w1115 w1118 T1 {"Left"=1240, "Top"=653} ("Position")] -> w1111
                          tunnel: [w1114 w1117 u16 26 ("estado")] -> w1110
                          tunnel: [w1116 w1119 w1122] -> w1109
                          tunnel: w1108 -> [w1116 w1119 w1123]
                          frame 1, Default {
                            # "accion no valida"
                            # "Torre 1"
                            n610 = local read "positionIncialDisco"() -> (w1115:T1)
                            n611 = local read "estado"() -> (w1114:u16)
                          }
                          frame 2 {
                            # "Volvio a la misma\nposicion"
                            # "Torre 2"
                            n612 = local read "positionIncialDisco"() -> (w1118:T1)
                            n613 = local read "estado"() -> (w1117:u16)
                          }
                          frame 3 {
                            # "Torre 3"
                            n614 = Increment(x=w1123) -> (x+1=w1122:i16)
                          }
                        }
                        n615 = local read "referenciaDisco"() -> (w1113:refnum<vi>)
                        n616 = local write "Tu numero de movimientos"(w1109) -> ()
                        n617 = property class="Bool (strict)"(reference=w1113, "Position"=w1111) -> ()  [unwired: 1 in, 2 out]
                      }
                    }
                  }
                }
              }
              frame 23 {
                # "Disco"
                # "Disco"
                # "Estado 23"
                n618 = local read "referenciaDisco"() -> (w1129:refnum<vi>)
                n619 = property class="Bool (strict)"(reference=w1129) -> ("Label.Text"=w1130:string)  [unwired: 1 in, 2 out]
                n620 = local read "Tu numero de movimientos"() -> (w1124:i16)
                n621 = Equal?(x=w1130, y="1") -> (x = y?=w1125:bool)
                n622 = Equal?(x=w1130, y="2") -> (x = y?=w1131:bool)
                n623 = Or(x=w1125, y=w1131) -> (x .or. y?=w1126:bool)
                n624 = case shown="True" w1126 {
                  tunnel: w1133 -> [_ w1138]
                  tunnel: [w1134 w1137] -> w1132
                  tunnel: w1125 -> [_ w1136]
                  tunnel: w1124 -> [_ w1135]
                  frame False {
                    n625 = local read "estado"() -> (w1134:u16)
                  }
                  frame True {
                    n626 = case shown="False" w1136 {
                      tunnel: w1138 -> [w1143 w1160]
                      tunnel: [w1141 w1158] -> w1137
                      tunnel: w1135 -> [w1139 w1156]
                      frame True {
                        # "Disco 1"
                        n627 = case shown="3" w1143 {
                          tunnel: [T1 {"Left"=223, "Top"=597} ("Position") T1 {"Left"=750, "Top"=597} ("Position") w1154] -> w1142
                          tunnel: [u16 22 ("estado") u16 16 ("estado") w1153] -> w1141
                          tunnel: [w1147 w1151 w1155] -> w1140
                          tunnel: w1139 -> [w1148 w1152 w1155]
                          frame 1, Default {
                            # "Torre 1"
                            n628 = Increment(x=w1148) -> (x+1=w1147:i16)
                          }
                          frame 2 {
                            # "Torre 2"
                            n629 = Increment(x=w1152) -> (x+1=w1151:i16)
                          }
                          frame 3 {
                            # "Volvio a la misma\nposicion"
                            # "Torre 3"
                            n630 = local read "positionIncialDisco"() -> (w1154:T1)
                            n631 = local read "estado"() -> (w1153:u16)
                          }
                        }
                        n632 = local read "referenciaDisco"() -> (w1144:refnum<vi>)
                        n633 = local write "Tu numero de movimientos"(w1140) -> ()
                        n634 = property class="Bool (strict)"(reference=w1144, "Position"=w1142) -> ()  [unwired: 1 in, 2 out]
                      }
                      frame False {
                        # "Disco 2"
                        n635 = case shown="3" w1160 {
                          tunnel: [w1163 T1 {"Left"=718, "Top"=597} ("positionIncialDisco") w1170] -> w1159
                          tunnel: [w1162 u16 21 ("estado") w1169] -> w1158
                          tunnel: [w1164 w1167 w1171] -> w1157
                          tunnel: w1156 -> [w1164 w1168 w1171]
                          frame 1, Default {
                            # "Volvio a la misma\nposicion"
                            # "Torre 1"
                            n636 = local read "positionIncialDisco"() -> (w1163:T1)
                            n637 = local read "estado"() -> (w1162:u16)
                          }
                          frame 2 {
                            # "Torre 2"
                            n638 = Increment(x=w1168) -> (x+1=w1167:i16)
                          }
                          frame 3 {
                            # "accion no valida"
                            # "Torre 3"
                            n639 = local read "positionIncialDisco"() -> (w1170:T1)
                            n640 = local read "estado"() -> (w1169:u16)
                          }
                        }
                        n641 = local read "referenciaDisco"() -> (w1161:refnum<vi>)
                        n642 = local write "Tu numero de movimientos"(w1157) -> ()
                        n643 = property class="Bool (strict)"(reference=w1161, "Position"=w1159) -> ()  [unwired: 1 in, 2 out]
                      }
                    }
                  }
                }
              }
              frame 24 {
                # "Disco"
                # "Disco"
                # "Estado 24"
                n644 = local read "referenciaDisco"() -> (w1177:refnum<vi>)
                n645 = property class="Bool (strict)"(reference=w1177) -> ("Label.Text"=w1178:string)  [unwired: 1 in, 2 out]
                n646 = local read "Tu numero de movimientos"() -> (w1172:i16)
                n647 = Equal?(x=w1178, y="1") -> (x = y?=w1173:bool)
                n648 = Equal?(x=w1178, y="2") -> (x = y?=w1179:bool)
                n649 = Or(x=w1173, y=w1179) -> (x .or. y?=w1174:bool)
                n650 = case shown="True" w1174 {
                  tunnel: w1181 -> [_ w1186]
                  tunnel: [w1182 w1185] -> w1180
                  tunnel: w1173 -> [_ w1184]
                  tunnel: w1172 -> [_ w1183]
                  frame False {
                    n651 = local read "estado"() -> (w1182:u16)
                  }
                  frame True {
                    n652 = case shown="False" w1184 {
                      tunnel: w1186 -> [w1191 w1208]
                      tunnel: [w1189 w1206] -> w1185
                      tunnel: w1183 -> [w1187 w1204]
                      frame True {
                        # "Disco 1"
                        n653 = case shown="3" w1191 {
                          tunnel: [T1 {"Left"=223, "Top"=653} ("Position") w1198 T1 {"Left"=1300, "Top"=541} ("Position")] -> w1190
                          tunnel: [u16 18 ("estado") w1197 u16 25 ("estado")] -> w1189
                          tunnel: [w1195 w1199 w1202] -> w1188
                          tunnel: w1187 -> [w1196 w1199 w1203]
                          frame 1, Default {
                            # "Torre 1"
                            n654 = Increment(x=w1196) -> (x+1=w1195:i16)
                          }
                          frame 2 {
                            # "Volvio a la misma\nposicion"
                            # "Torre 2"
                            n655 = local read "positionIncialDisco"() -> (w1198:T1)
                            n656 = local read "estado"() -> (w1197:u16)
                          }
                          frame 3 {
                            # "Torre 3"
                            n657 = Increment(x=w1203) -> (x+1=w1202:i16)
                          }
                        }
                        n658 = local read "referenciaDisco"() -> (w1192:refnum<vi>)
                        n659 = local write "Tu numero de movimientos"(w1188) -> ()
                        n660 = property class="Bool (strict)"(reference=w1192, "Position"=w1190) -> ()  [unwired: 1 in, 2 out]
                      }
                      frame False {
                        # "Disco 2"
                        n661 = case shown="1, Default" w1208 {
                          tunnel: [T1 {"Left"=193, "Top"=653} ("Position") w1215 w1218] -> w1207
                          tunnel: [u16 27 ("estado") w1214 w1217] -> w1206
                          tunnel: [w1212 w1216 w1219] -> w1205
                          tunnel: w1204 -> [w1213 w1216 w1219]
                          frame 1, Default {
                            # "Torre 1"
                            n662 = Increment(x=w1213) -> (x+1=w1212:i16)
                          }
                          frame 2 {
                            # "accion no valida"
                            # "Torre 2"
                            n663 = local read "positionIncialDisco"() -> (w1215:T1)
                            n664 = local read "estado"() -> (w1214:u16)
                          }
                          frame 3 {
                            # "Volvio a la misma\nposicion"
                            # "accion no valida"
                            # "Torre 3"
                            n665 = local read "positionIncialDisco"() -> (w1218:T1)
                            n666 = local read "estado"() -> (w1217:u16)
                          }
                        }
                        n667 = local read "referenciaDisco"() -> (w1209:refnum<vi>)
                        n668 = local write "Tu numero de movimientos"(w1205) -> ()
                        n669 = property class="Bool (strict)"(reference=w1209, "Position"=w1207) -> ()  [unwired: 1 in, 2 out]
                      }
                    }
                  }
                }
              }
              frame 25 {
                # "Disco"
                # "Disco"
                # "Estado 25"
                n670 = local read "referenciaDisco"() -> (w1225:refnum<vi>)
                n671 = property class="Bool (strict)"(reference=w1225) -> ("Label.Text"=w1226:string)  [unwired: 1 in, 2 out]
                n672 = local read "Tu numero de movimientos"() -> (w1220:i16)
                n673 = Equal?(x=w1226, y="1") -> (x = y?=w1221:bool)
                n674 = Equal?(x=w1226, y="1") -> (x = y?=w1227:bool)
                n675 = Or(x=w1221, y=w1227) -> (x .or. y?=w1222:bool)
                n676 = case shown="True" w1222 {
                  tunnel: w1229 -> [_ w1236]
                  tunnel: [w1230 w1235] -> w1228
                  tunnel: w1221 -> [_ _]
                  tunnel: w1220 -> [_ w1234]
                  frame False {
                    n677 = local read "estado"() -> (w1230:u16)
                  }
                  frame True {
                    # "Disco 1"
                    n678 = case shown="3" w1236 {
                      tunnel: [T1 {"Left"=223, "Top"=653} ("Position") T1 {"Left"=750, "Top"=653} ("Position") w1246] -> w1232
                      tunnel: [u16 18 ("estado") u16 24 ("estado") w1245] -> w1235
                      tunnel: [w1239 w1242 w1247] -> w1231
                      tunnel: w1234 -> [w1240 w1244 w1247]
                      frame 1, Default {
                        # "Torre 1"
                        n679 = Increment(x=w1240) -> (x+1=w1239:i16)
                      }
                      frame 2 {
                        # "Torre 2"
                        n680 = Increment(x=w1244) -> (x+1=w1242:i16)
                      }
                      frame 3 {
                        # "Volvio a la misma\nposicion"
                        # "Torre 3"
                        n681 = local read "positionIncialDisco"() -> (w1246:T1)
                        n682 = local read "estado"() -> (w1245:u16)
                      }
                    }
                    n683 = local read "referenciaDisco"() -> (w1233:refnum<vi>)
                    n684 = local write "Tu numero de movimientos"(w1231) -> ()
                    n685 = property class="Bool (strict)"(reference=w1233, "Position"=w1232) -> ()  [unwired: 1 in, 2 out]
                  }
                }
              }
              frame 26 {
                # "Disco"
                # "Disco"
                # "Estado 26"
                n686 = local read "referenciaDisco"() -> (w1253:refnum<vi>)
                n687 = property class="Bool (strict)"(reference=w1253) -> ("Label.Text"=w1254:string)  [unwired: 1 in, 2 out]
                n688 = local read "Tu numero de movimientos"() -> (w1248:i16)
                n689 = Equal?(x=w1254, y="1") -> (x = y?=w1249:bool)
                n690 = Equal?(x=w1254, y="3") -> (x = y?=w1255:bool)
                n691 = Or(x=w1249, y=w1255) -> (x .or. y?=w1250:bool)
                n692 = case shown="True" w1250 {
                  tunnel: w1257 -> [_ w1262]
                  tunnel: [w1258 w1261] -> w1256
                  tunnel: w1249 -> [_ w1260]
                  tunnel: w1248 -> [_ w1259]
                  frame False {
                    n693 = local read "estado"() -> (w1258:u16)
                  }
                  frame True {
                    n694 = case shown="False" w1260 {
                      tunnel: w1262 -> [w1267 w1284]
                      tunnel: [w1265 w1282] -> w1261
                      tunnel: w1259 -> [w1263 w1280]
                      frame True {
                        # "Disco 1"
                        n695 = case shown="1, Default" w1267 {
                          tunnel: [w1270 T1 {"Left"=750, "Top"=653} ("Position") T1 {"Left"=1300, "Top"=597} ("Position")] -> w1266
                          tunnel: [w1269 u16 27 ("estado") u16 19 ("estado")] -> w1265
                          tunnel: [w1271 w1274 w1278] -> w1264
                          tunnel: w1263 -> [w1271 w1275 w1279]
                          frame 1, Default {
                            # "Volvio a la misma\nposicion"
                            # "Torre 1"
                            n696 = local read "positionIncialDisco"() -> (w1270:T1)
                            n697 = local read "estado"() -> (w1269:u16)
                          }
                          frame 2 {
                            # "Torre 2"
                            n698 = Increment(x=w1275) -> (x+1=w1274:i16)
                          }
                          frame 3 {
                            # "Torre 3"
                            n699 = Increment(x=w1279) -> (x+1=w1278:i16)
                          }
                        }
                        n700 = local read "referenciaDisco"() -> (w1268:refnum<vi>)
                        n701 = local write "Tu numero de movimientos"(w1264) -> ()
                        n702 = property class="Bool (strict)"(reference=w1268, "Position"=w1266) -> ()  [unwired: 1 in, 2 out]
                      }
                      frame False {
                        # "Disco 3"
                        n703 = case shown="3" w1284 {
                          tunnel: [w1287 T1 {"Left"=690, "Top"=653} ("Position") w1294] -> w1283
                          tunnel: [w1286 u16 22 ("estado") w1293] -> w1282
                          tunnel: [w1288 w1290 w1295] -> w1281
                          tunnel: w1280 -> [w1288 w1292 w1295]
                          frame 1, Default {
                            # "accion no valida"
                            # "Torre 1"
                            n704 = local read "positionIncialDisco"() -> (w1287:T1)
                            n705 = local read "estado"() -> (w1286:u16)
                          }
                          frame 2 {
                            # "Torre 2"
                            n706 = Increment(x=w1292) -> (x+1=w1290:i16)
                          }
                          frame 3 {
                            # "Volvio a la misma\nposicion"
                            # "Torre 3"
                            n707 = local read "positionIncialDisco"() -> (w1294:T1)
                            n708 = local read "estado"() -> (w1293:u16)
                          }
                        }
                        n709 = local read "referenciaDisco"() -> (w1285:refnum<vi>)
                        n710 = local write "Tu numero de movimientos"(w1281) -> ()
                        n711 = property class="Bool (strict)"(reference=w1285, "Position"=w1283) -> ()  [unwired: 1 in, 2 out]
                      }
                    }
                  }
                }
              }
              frame 27 {
                # "Disco"
                # "Disco"
                # "Estado 27"
                n712 = local read "referenciaDisco"() -> (w1301:refnum<vi>)
                n713 = property class="Bool (strict)"(reference=w1301) -> ("Label.Text"=w1302:string)  [unwired: 1 in, 2 out]
                n714 = local read "Tu numero de movimientos"() -> (w1296:i16)
                n715 = Equal?(x=w1302, y="1") -> (x = y?=w1297:bool)
                n716 = Equal?(x=w1302, y="2") -> (x = y?=w1303:bool)
                n717 = Or(x=w1297, y=w1303) -> (x .or. y?=w1298:bool)
                n718 = case shown="True" w1298 {
                  tunnel: w1305 -> [_ w1310]
                  tunnel: [w1306 w1309] -> w1304
                  tunnel: w1297 -> [_ w1308]
                  tunnel: w1296 -> [_ w1307]
                  frame False {
                    n719 = local read "estado"() -> (w1306:u16)
                  }
                  frame True {
                    n720 = case shown="False" w1308 {
                      tunnel: w1310 -> [w1315 w1332]
                      tunnel: [w1313 w1330] -> w1309
                      tunnel: w1307 -> [w1311 w1328]
                      frame True {
                        # "Disco 1"
                        n721 = case shown="3" w1315 {
                          tunnel: [T1 {"Left"=223, "Top"=597} ("Position") w1322 T1 {"Left"=1300, "Top"=597} ("Position")] -> w1314
                          tunnel: [u16 26 ("estado") w1321 u16 19 ("estado")] -> w1313
                          tunnel: [w1319 w1323 w1326] -> w1312
                          tunnel: w1311 -> [w1320 w1323 w1327]
                          frame 1, Default {
                            # "Torre 1"
                            n722 = Increment(x=w1320) -> (x+1=w1319:i16)
                          }
                          frame 2 {
                            # "Volvio a la misma\nposicion"
                            # "Torre 2"
                            n723 = local read "positionIncialDisco"() -> (w1322:T1)
                            n724 = local read "estado"() -> (w1321:u16)
                          }
                          frame 3 {
                            # "Torre 3"
                            n725 = Increment(x=w1327) -> (x+1=w1326:i16)
                          }
                        }
                        n726 = local read "referenciaDisco"() -> (w1316:refnum<vi>)
                        n727 = local write "Tu numero de movimientos"(w1312) -> ()
                        n728 = property class="Bool (strict)"(reference=w1316, "Position"=w1314) -> ()  [unwired: 1 in, 2 out]
                      }
                      frame False {
                        # "Disco 2"
                        n729 = case shown="3" w1332 {
                          tunnel: [w1335 w1337 T1 {"Left"=1270, "Top"=597} ("Position")] -> w1331
                          tunnel: [w1334 w1338 u16 24 ("estado")] -> w1330
                          tunnel: [w1336 w1339 w1340] -> w1329
                          tunnel: w1328 -> [w1336 w1339 w1343]
                          frame 1, Default {
                            # "Volvio a la misma\nposicion"
                            # "Torre 1"
                            n730 = local read "positionIncialDisco"() -> (w1335:T1)
                            n731 = local read "estado"() -> (w1334:u16)
                          }
                          frame 2 {
                            # "accion no valida"
                            # "Torre 2"
                            n732 = local read "positionIncialDisco"() -> (w1337:T1)
                            n733 = local read "estado"() -> (w1338:u16)
                          }
                          frame 3 {
                            # "Torre 3"
                            n734 = Increment(x=w1343) -> (x+1=w1340:i16)
                          }
                        }
                        n735 = local read "referenciaDisco"() -> (w1333:refnum<vi>)
                        n736 = local write "Tu numero de movimientos"(w1329) -> ()
                        n737 = property class="Bool (strict)"(reference=w1333, "Position"=w1331) -> ()  [unwired: 1 in, 2 out]
                      }
                    }
                  }
                }
              }
            }
            n738 = local write "estado"(w57) -> ()
          }
        }
      }
      frame 3 {
        # "El mouse esta sostenido por el usuario"
        n739 = local read "estado"() -> (w1344:u16)
        n740 = case shown="1" w1344 {
          frame 0, Default {
            # "Estado 0"
            # "Disco"
            # "Disco"
            n741 = local read "referenciaDisco"() -> (w1348:refnum<vi>)
            n742 = property class="Bool (strict)"(reference=w1348) -> ("Label.Text"=w1349:string)  [unwired: 1 in, 2 out]
            n743 = Equal?(x=w1349, y="1") -> (x = y?=w1351:bool)
            n744 = Equal?(x=w1349, y="1") -> (x = y?=w1350:bool)
            n745 = Or(x=w1351, y=w1350) -> (x .or. y?=w1345:bool)
            n746 = case shown="True" w1345 {
              frame False {
              }
              frame True {
                n747 = local read "referenciaDisco"() -> (w1355:refnum<vi>)
                n748 = local read "coordenadas del mouse"() -> (w1354:T2)
                n749 = property class="Bool (strict)"(reference=w1355) -> (reference out=w1358:refnum<vi>, "Bounds"=w1356:T3)  [unwired: 1 in, 1 out]
                n750 = Divide(x=w1356, y=T3 {"Width"=2, "Height"=2}) -> (x/y=w1353:cluster{"Width":dbl, "Height":dbl})
                n751 = Subtract(x=w1354, y=w1353) -> (x-y=w1357:cluster{dbl, dbl})
                n752 = property class="Bool (strict)"(reference=w1358, "Position"=w1357) -> ()  [unwired: 1 in, 2 out]
              }
            }
          }
          frame 1 {
            # "Estado 1"
            # "Disco"
            # "Disco"
            n753 = local read "referenciaDisco"() -> (w1362:refnum<vi>)
            n754 = property class="Bool (strict)"(reference=w1362) -> ("Label.Text"=w1363:string)  [unwired: 1 in, 2 out]
            n755 = Equal?(x=w1363, y="1") -> (x = y?=w1365:bool)
            n756 = Equal?(x=w1363, y="2") -> (x = y?=w1364:bool)
            n757 = Or(x=w1365, y=w1364) -> (x .or. y?=w1359:bool)
            n758 = case shown="True" w1359 {
              frame False {
              }
              frame True {
                n759 = local read "referenciaDisco"() -> (w1369:refnum<vi>)
                n760 = local read "coordenadas del mouse"() -> (w1368:T2)
                n761 = property class="Bool (strict)"(reference=w1369) -> (reference out=w1372:refnum<vi>, "Bounds"=w1370:T3)  [unwired: 1 in, 1 out]
                n762 = Divide(x=w1370, y=T3 {"Width"=2, "Height"=2}) -> (x/y=w1367:cluster{"Width":dbl, "Height":dbl})
                n763 = Subtract(x=w1368, y=w1367) -> (x-y=w1371:cluster{dbl, dbl})
                n764 = property class="Bool (strict)"(reference=w1372, "Position"=w1371) -> ()  [unwired: 1 in, 2 out]
              }
            }
          }
          frame 2 {
            # "Estado 2"
            # "Disco"
            # "Disco"
            n765 = local read "referenciaDisco"() -> (w1376:refnum<vi>)
            n766 = property class="Bool (strict)"(reference=w1376) -> ("Label.Text"=w1377:string)  [unwired: 1 in, 2 out]
            n767 = Equal?(x=w1377, y="1") -> (x = y?=w1379:bool)
            n768 = Equal?(x=w1377, y="2") -> (x = y?=w1378:bool)
            n769 = Or(x=w1379, y=w1378) -> (x .or. y?=w1373:bool)
            n770 = case shown="True" w1373 {
              frame False {
              }
              frame True {
                n771 = local read "referenciaDisco"() -> (w1383:refnum<vi>)
                n772 = local read "coordenadas del mouse"() -> (w1382:T2)
                n773 = property class="Bool (strict)"(reference=w1383) -> (reference out=w1386:refnum<vi>, "Bounds"=w1384:T3)  [unwired: 1 in, 1 out]
                n774 = Divide(x=w1384, y=T3 {"Width"=2, "Height"=2}) -> (x/y=w1381:cluster{"Width":dbl, "Height":dbl})
                n775 = Subtract(x=w1382, y=w1381) -> (x-y=w1385:cluster{dbl, dbl})
                n776 = property class="Bool (strict)"(reference=w1386, "Position"=w1385) -> ()  [unwired: 1 in, 2 out]
              }
            }
          }
          frame 3 {
            # "Estado 3"
            # "Disco"
            # "Disco"
            n777 = local read "referenciaDisco"() -> (w1390:refnum<vi>)
            n778 = property class="Bool (strict)"(reference=w1390) -> ("Label.Text"=w1391:string)  [unwired: 1 in, 2 out]
            n779 = Equal?(x=w1391, y="1") -> (x = y?=w1393:bool)
            n780 = Equal?(x=w1391, y="2") -> (x = y?=w1392:bool)
            n781 = Or(x=w1393, y=w1392) -> (x .or. y?=w1387:bool)
            n782 = case shown="True" w1387 {
              frame False {
              }
              frame True {
                n783 = local read "referenciaDisco"() -> (w1397:refnum<vi>)
                n784 = local read "coordenadas del mouse"() -> (w1396:T2)
                n785 = property class="Bool (strict)"(reference=w1397) -> (reference out=w1400:refnum<vi>, "Bounds"=w1398:T3)  [unwired: 1 in, 1 out]
                n786 = Divide(x=w1398, y=T3 {"Width"=2, "Height"=2}) -> (x/y=w1395:cluster{"Width":dbl, "Height":dbl})
                n787 = Subtract(x=w1396, y=w1395) -> (x-y=w1399:cluster{dbl, dbl})
                n788 = property class="Bool (strict)"(reference=w1400, "Position"=w1399) -> ()  [unwired: 1 in, 2 out]
              }
            }
          }
          frame 4 {
            # "Estado 4"
            # "Disco"
            # "Disco"
            n789 = local read "referenciaDisco"() -> (w1404:refnum<vi>)
            n790 = property class="Bool (strict)"(reference=w1404) -> ("Label.Text"=w1405:string)  [unwired: 1 in, 2 out]
            n791 = Equal?(x=w1405, y="1") -> (x = y?=w1407:bool)
            n792 = Equal?(x=w1405, y="2") -> (x = y?=w1406:bool)
            n793 = Or(x=w1407, y=w1406) -> (x .or. y?=w1401:bool)
            n794 = case shown="True" w1401 {
              frame False {
              }
              frame True {
                n795 = local read "referenciaDisco"() -> (w1411:refnum<vi>)
                n796 = local read "coordenadas del mouse"() -> (w1410:T2)
                n797 = property class="Bool (strict)"(reference=w1411) -> (reference out=w1414:refnum<vi>, "Bounds"=w1412:T3)  [unwired: 1 in, 1 out]
                n798 = Divide(x=w1412, y=T3 {"Width"=2, "Height"=2}) -> (x/y=w1409:cluster{"Width":dbl, "Height":dbl})
                n799 = Subtract(x=w1410, y=w1409) -> (x-y=w1413:cluster{dbl, dbl})
                n800 = property class="Bool (strict)"(reference=w1414, "Position"=w1413) -> ()  [unwired: 1 in, 2 out]
              }
            }
          }
          frame 5 {
            # "Estado 5"
            # "Disco"
            # "Disco"
            n801 = local read "referenciaDisco"() -> (w1418:refnum<vi>)
            n802 = property class="Bool (strict)"(reference=w1418) -> ("Label.Text"=w1419:string)  [unwired: 1 in, 2 out]
            n803 = Equal?(x=w1419, y="1") -> (x = y?=w1421:bool)
            n804 = Equal?(x=w1419, y="2") -> (x = y?=w1420:bool)
            n805 = Or(x=w1421, y=w1420) -> (x .or. y?=w1415:bool)
            n806 = case shown="True" w1415 {
              frame False {
              }
              frame True {
                n807 = local read "referenciaDisco"() -> (w1425:refnum<vi>)
                n808 = local read "coordenadas del mouse"() -> (w1424:T2)
                n809 = property class="Bool (strict)"(reference=w1425) -> (reference out=w1428:refnum<vi>, "Bounds"=w1426:T3)  [unwired: 1 in, 1 out]
                n810 = Divide(x=w1426, y=T3 {"Width"=2, "Height"=2}) -> (x/y=w1423:cluster{"Width":dbl, "Height":dbl})
                n811 = Subtract(x=w1424, y=w1423) -> (x-y=w1427:cluster{dbl, dbl})
                n812 = property class="Bool (strict)"(reference=w1428, "Position"=w1427) -> ()  [unwired: 1 in, 2 out]
              }
            }
          }
          frame 6 {
            # "Estado 6"
            # "Disco"
            # "Disco"
            n813 = local read "referenciaDisco"() -> (w1432:refnum<vi>)
            n814 = property class="Bool (strict)"(reference=w1432) -> ("Label.Text"=w1433:string)  [unwired: 1 in, 2 out]
            n815 = Equal?(x=w1433, y="1") -> (x = y?=w1435:bool)
            n816 = Equal?(x=w1433, y="3") -> (x = y?=w1434:bool)
            n817 = Or(x=w1435, y=w1434) -> (x .or. y?=w1429:bool)
            n818 = case shown="True" w1429 {
              frame False {
              }
              frame True {
                n819 = local read "referenciaDisco"() -> (w1439:refnum<vi>)
                n820 = local read "coordenadas del mouse"() -> (w1438:T2)
                n821 = property class="Bool (strict)"(reference=w1439) -> (reference out=w1442:refnum<vi>, "Bounds"=w1440:T3)  [unwired: 1 in, 1 out]
                n822 = Divide(x=w1440, y=T3 {"Width"=2, "Height"=2}) -> (x/y=w1437:cluster{"Width":dbl, "Height":dbl})
                n823 = Subtract(x=w1438, y=w1437) -> (x-y=w1441:cluster{dbl, dbl})
                n824 = property class="Bool (strict)"(reference=w1442, "Position"=w1441) -> ()  [unwired: 1 in, 2 out]
              }
            }
          }
          frame 7 {
            # "Estado 7"
            # "Disco"
            # "Disco"
            n825 = local read "referenciaDisco"() -> (w1446:refnum<vi>)
            n826 = property class="Bool (strict)"(reference=w1446) -> ("Label.Text"=w1447:string)  [unwired: 1 in, 2 out]
            n827 = Equal?(x=w1447, y="1") -> (x = y?=w1449:bool)
            n828 = Equal?(x=w1447, y="2") -> (x = y?=w1448:bool)
            n829 = Or(x=w1449, y=w1448) -> (x .or. y?=w1443:bool)
            n830 = case shown="True" w1443 {
              frame False {
              }
              frame True {
                n831 = local read "referenciaDisco"() -> (w1453:refnum<vi>)
                n832 = local read "coordenadas del mouse"() -> (w1452:T2)
                n833 = property class="Bool (strict)"(reference=w1453) -> (reference out=w1456:refnum<vi>, "Bounds"=w1454:T3)  [unwired: 1 in, 1 out]
                n834 = Divide(x=w1454, y=T3 {"Width"=2, "Height"=2}) -> (x/y=w1451:cluster{"Width":dbl, "Height":dbl})
                n835 = Subtract(x=w1452, y=w1451) -> (x-y=w1455:cluster{dbl, dbl})
                n836 = property class="Bool (strict)"(reference=w1456, "Position"=w1455) -> ()  [unwired: 1 in, 2 out]
              }
            }
          }
          frame 8 {
            # "Estado 8"
            # "Disco"
            # "Disco"
            n837 = local read "referenciaDisco"() -> (w1460:refnum<vi>)
            n838 = property class="Bool (strict)"(reference=w1460) -> ("Label.Text"=w1461:string)  [unwired: 1 in, 2 out]
            n839 = Equal?(x=w1461, y="1") -> (x = y?=w1463:bool)
            n840 = Equal?(x=w1461, y="3") -> (x = y?=w1462:bool)
            n841 = Or(x=w1463, y=w1462) -> (x .or. y?=w1457:bool)
            n842 = case shown="True" w1457 {
              frame False {
              }
              frame True {
                n843 = local read "referenciaDisco"() -> (w1467:refnum<vi>)
                n844 = local read "coordenadas del mouse"() -> (w1466:T2)
                n845 = property class="Bool (strict)"(reference=w1467) -> (reference out=w1470:refnum<vi>, "Bounds"=w1468:T3)  [unwired: 1 in, 1 out]
                n846 = Divide(x=w1468, y=T3 {"Width"=2, "Height"=2}) -> (x/y=w1465:cluster{"Width":dbl, "Height":dbl})
                n847 = Subtract(x=w1466, y=w1465) -> (x-y=w1469:cluster{dbl, dbl})
                n848 = property class="Bool (strict)"(reference=w1470, "Position"=w1469) -> ()  [unwired: 1 in, 2 out]
              }
            }
          }
          frame 9 {
            # "Estado 9"
            # "Disco"
            # "Disco"
            n849 = local read "referenciaDisco"() -> (w1474:refnum<vi>)
            n850 = property class="Bool (strict)"(reference=w1474) -> ("Label.Text"=w1475:string)  [unwired: 1 in, 2 out]
            n851 = Equal?(x=w1475, y="1") -> (x = y?=w1477:bool)
            n852 = Equal?(x=w1475, y="3") -> (x = y?=w1476:bool)
            n853 = Or(x=w1477, y=w1476) -> (x .or. y?=w1471:bool)
            n854 = case shown="True" w1471 {
              frame False {
              }
              frame True {
                n855 = local read "referenciaDisco"() -> (w1481:refnum<vi>)
                n856 = local read "coordenadas del mouse"() -> (w1480:T2)
                n857 = property class="Bool (strict)"(reference=w1481) -> (reference out=w1484:refnum<vi>, "Bounds"=w1482:T3)  [unwired: 1 in, 1 out]
                n858 = Divide(x=w1482, y=T3 {"Width"=2, "Height"=2}) -> (x/y=w1479:cluster{"Width":dbl, "Height":dbl})
                n859 = Subtract(x=w1480, y=w1479) -> (x-y=w1483:cluster{dbl, dbl})
                n860 = property class="Bool (strict)"(reference=w1484, "Position"=w1483) -> ()  [unwired: 1 in, 2 out]
              }
            }
          }
          frame 10 {
            # "Estado 10"
            # "Disco"
            # "Disco"
            n861 = local read "referenciaDisco"() -> (w1488:refnum<vi>)
            n862 = property class="Bool (strict)"(reference=w1488) -> ("Label.Text"=w1489:string)  [unwired: 1 in, 2 out]
            n863 = Equal?(x=w1489, y="1") -> (x = y?=w1491:bool)
            n864 = Equal?(x=w1489, y="3") -> (x = y?=w1490:bool)
            n865 = Or(x=w1491, y=w1490) -> (x .or. y?=w1485:bool)
            n866 = case shown="True" w1485 {
              frame False {
              }
              frame True {
                n867 = local read "referenciaDisco"() -> (w1495:refnum<vi>)
                n868 = local read "coordenadas del mouse"() -> (w1494:T2)
                n869 = property class="Bool (strict)"(reference=w1495) -> (reference out=w1498:refnum<vi>, "Bounds"=w1496:T3)  [unwired: 1 in, 1 out]
                n870 = Divide(x=w1496, y=T3 {"Width"=2, "Height"=2}) -> (x/y=w1493:cluster{"Width":dbl, "Height":dbl})
                n871 = Subtract(x=w1494, y=w1493) -> (x-y=w1497:cluster{dbl, dbl})
                n872 = property class="Bool (strict)"(reference=w1498, "Position"=w1497) -> ()  [unwired: 1 in, 2 out]
              }
            }
          }
          frame 11 {
            # "Estado 11"
            # "Disco"
            # "Disco"
            n873 = local read "referenciaDisco"() -> (w1502:refnum<vi>)
            n874 = property class="Bool (strict)"(reference=w1502) -> ("Label.Text"=w1503:string)  [unwired: 1 in, 2 out]
            n875 = Equal?(x=w1503, y="1") -> (x = y?=w1505:bool)
            n876 = Equal?(x=w1503, y="2") -> (x = y?=w1504:bool)
            n877 = Or(x=w1505, y=w1504) -> (x .or. y?=w1499:bool)
            n878 = case shown="True" w1499 {
              frame False {
              }
              frame True {
                n879 = local read "referenciaDisco"() -> (w1509:refnum<vi>)
                n880 = local read "coordenadas del mouse"() -> (w1508:T2)
                n881 = property class="Bool (strict)"(reference=w1509) -> (reference out=w1512:refnum<vi>, "Bounds"=w1510:T3)  [unwired: 1 in, 1 out]
                n882 = Divide(x=w1510, y=T3 {"Width"=2, "Height"=2}) -> (x/y=w1507:cluster{"Width":dbl, "Height":dbl})
                n883 = Subtract(x=w1508, y=w1507) -> (x-y=w1511:cluster{dbl, dbl})
                n884 = property class="Bool (strict)"(reference=w1512, "Position"=w1511) -> ()  [unwired: 1 in, 2 out]
              }
            }
          }
          frame 12 {
            # "Estado 12"
            # "Disco"
            # "Disco"
            n885 = local read "referenciaDisco"() -> (w1516:refnum<vi>)
            n886 = property class="Bool (strict)"(reference=w1516) -> ("Label.Text"=w1517:string)  [unwired: 1 in, 2 out]
            n887 = Equal?(x=w1517, y="1") -> (x = y?=w1519:bool)
            n888 = Equal?(x=w1517, y="2") -> (x = y?=w1518:bool)
            n889 = Or(x=w1519, y=w1518) -> (x .or. y?=w1513:bool)
            n890 = case shown="True" w1513 {
              frame False {
              }
              frame True {
                n891 = local read "referenciaDisco"() -> (w1523:refnum<vi>)
                n892 = local read "coordenadas del mouse"() -> (w1522:T2)
                n893 = property class="Bool (strict)"(reference=w1523) -> (reference out=w1526:refnum<vi>, "Bounds"=w1524:T3)  [unwired: 1 in, 1 out]
                n894 = Divide(x=w1524, y=T3 {"Width"=2, "Height"=2}) -> (x/y=w1521:cluster{"Width":dbl, "Height":dbl})
                n895 = Subtract(x=w1522, y=w1521) -> (x-y=w1525:cluster{dbl, dbl})
                n896 = property class="Bool (strict)"(reference=w1526, "Position"=w1525) -> ()  [unwired: 1 in, 2 out]
              }
            }
          }
          frame 13 {
            # "Estado 13"
            # "Disco"
            # "Disco"
            n897 = local read "referenciaDisco"() -> (w1530:refnum<vi>)
            n898 = property class="Bool (strict)"(reference=w1530) -> ("Label.Text"=w1531:string)  [unwired: 1 in, 2 out]
            n899 = Equal?(x=w1531, y="1") -> (x = y?=w1533:bool)
            n900 = Equal?(x=w1531, y="2") -> (x = y?=w1532:bool)
            n901 = Or(x=w1533, y=w1532) -> (x .or. y?=w1527:bool)
            n902 = case shown="True" w1527 {
              frame False {
              }
              frame True {
                n903 = local read "referenciaDisco"() -> (w1537:refnum<vi>)
                n904 = local read "coordenadas del mouse"() -> (w1536:T2)
                n905 = property class="Bool (strict)"(reference=w1537) -> (reference out=w1540:refnum<vi>, "Bounds"=w1538:T3)  [unwired: 1 in, 1 out]
                n906 = Divide(x=w1538, y=T3 {"Width"=2, "Height"=2}) -> (x/y=w1535:cluster{"Width":dbl, "Height":dbl})
                n907 = Subtract(x=w1536, y=w1535) -> (x-y=w1539:cluster{dbl, dbl})
                n908 = property class="Bool (strict)"(reference=w1540, "Position"=w1539) -> ()  [unwired: 1 in, 2 out]
              }
            }
          }
          frame 14 {
            # "Estado 14"
            # "Disco"
            # "Disco"
            n909 = local read "referenciaDisco"() -> (w1544:refnum<vi>)
            n910 = property class="Bool (strict)"(reference=w1544) -> ("Label.Text"=w1545:string)  [unwired: 1 in, 2 out]
            n911 = Equal?(x=w1545, y="1") -> (x = y?=w1547:bool)
            n912 = Equal?(x=w1545, y="2") -> (x = y?=w1546:bool)
            n913 = Or(x=w1547, y=w1546) -> (x .or. y?=w1541:bool)
            n914 = case shown="True" w1541 {
              frame False {
              }
              frame True {
                n915 = local read "referenciaDisco"() -> (w1551:refnum<vi>)
                n916 = local read "coordenadas del mouse"() -> (w1550:T2)
                n917 = property class="Bool (strict)"(reference=w1551) -> (reference out=w1554:refnum<vi>, "Bounds"=w1552:T3)  [unwired: 1 in, 1 out]
                n918 = Divide(x=w1552, y=T3 {"Width"=2, "Height"=2}) -> (x/y=w1549:cluster{"Width":dbl, "Height":dbl})
                n919 = Subtract(x=w1550, y=w1549) -> (x-y=w1553:cluster{dbl, dbl})
                n920 = property class="Bool (strict)"(reference=w1554, "Position"=w1553) -> ()  [unwired: 1 in, 2 out]
              }
            }
          }
          frame 15 {
            # "Estado 15"
            # "Disco"
            # "Disco"
            n921 = local read "referenciaDisco"() -> (w1558:refnum<vi>)
            n922 = property class="Bool (strict)"(reference=w1558) -> ("Label.Text"=w1559:string)  [unwired: 1 in, 2 out]
            n923 = Equal?(x=w1559, y="1") -> (x = y?=w1561:bool)
            n924 = Equal?(x=w1559, y="2") -> (x = y?=w1560:bool)
            n925 = Or(x=w1561, y=w1560) -> (x .or. y?=w1555:bool)
            n926 = case shown="True" w1555 {
              frame False {
              }
              frame True {
                n927 = local read "referenciaDisco"() -> (w1565:refnum<vi>)
                n928 = local read "coordenadas del mouse"() -> (w1564:T2)
                n929 = property class="Bool (strict)"(reference=w1565) -> (reference out=w1568:refnum<vi>, "Bounds"=w1566:T3)  [unwired: 1 in, 1 out]
                n930 = Divide(x=w1566, y=T3 {"Width"=2, "Height"=2}) -> (x/y=w1563:cluster{"Width":dbl, "Height":dbl})
                n931 = Subtract(x=w1564, y=w1563) -> (x-y=w1567:cluster{dbl, dbl})
                n932 = property class="Bool (strict)"(reference=w1568, "Position"=w1567) -> ()  [unwired: 1 in, 2 out]
              }
            }
          }
          frame 16 {
            # "Estado 16"
            # "Disco"
            # "Disco"
            n933 = local read "referenciaDisco"() -> (w1572:refnum<vi>)
            n934 = property class="Bool (strict)"(reference=w1572) -> ("Label.Text"=w1573:string)  [unwired: 1 in, 2 out]
            n935 = Equal?(x=w1573, y="1") -> (x = y?=w1575:bool)
            n936 = Equal?(x=w1573, y="2") -> (x = y?=w1574:bool)
            n937 = Or(x=w1575, y=w1574) -> (x .or. y?=w1569:bool)
            n938 = case shown="True" w1569 {
              frame False {
              }
              frame True {
                n939 = local read "referenciaDisco"() -> (w1579:refnum<vi>)
                n940 = local read "coordenadas del mouse"() -> (w1578:T2)
                n941 = property class="Bool (strict)"(reference=w1579) -> (reference out=w1582:refnum<vi>, "Bounds"=w1580:T3)  [unwired: 1 in, 1 out]
                n942 = Divide(x=w1580, y=T3 {"Width"=2, "Height"=2}) -> (x/y=w1577:cluster{"Width":dbl, "Height":dbl})
                n943 = Subtract(x=w1578, y=w1577) -> (x-y=w1581:cluster{dbl, dbl})
                n944 = property class="Bool (strict)"(reference=w1582, "Position"=w1581) -> ()  [unwired: 1 in, 2 out]
              }
            }
          }
          frame 17 {
            # "Estado 17\nes igual al Estado 10"
            # "Disco"
            # "Disco"
            n945 = local read "referenciaDisco"() -> (w1586:refnum<vi>)
            n946 = property class="Bool (strict)"(reference=w1586) -> ("Label.Text"=w1587:string)  [unwired: 1 in, 2 out]
            n947 = Equal?(x=w1587, y="1") -> (x = y?=w1589:bool)
            n948 = Equal?(x=w1587, y="2") -> (x = y?=w1588:bool)
            n949 = Or(x=w1589, y=w1588) -> (x .or. y?=w1583:bool)
            n950 = case shown="True" w1583 {
              frame False {
              }
              frame True {
                n951 = local read "referenciaDisco"() -> (w1593:refnum<vi>)
                n952 = local read "coordenadas del mouse"() -> (w1592:T2)
                n953 = property class="Bool (strict)"(reference=w1593) -> (reference out=w1596:refnum<vi>, "Bounds"=w1594:T3)  [unwired: 1 in, 1 out]
                n954 = Divide(x=w1594, y=T3 {"Width"=2, "Height"=2}) -> (x/y=w1591:cluster{"Width":dbl, "Height":dbl})
                n955 = Subtract(x=w1592, y=w1591) -> (x-y=w1595:cluster{dbl, dbl})
                n956 = property class="Bool (strict)"(reference=w1596, "Position"=w1595) -> ()  [unwired: 1 in, 2 out]
              }
            }
          }
          frame 18 {
            # "Estado 18"
            # "Disco"
            # "Disco"
            n957 = local read "referenciaDisco"() -> (w1600:refnum<vi>)
            n958 = property class="Bool (strict)"(reference=w1600) -> ("Label.Text"=w1601:string)  [unwired: 1 in, 2 out]
            n959 = Equal?(x=w1601, y="1") -> (x = y?=w1603:bool)
            n960 = Equal?(x=w1601, y="2") -> (x = y?=w1602:bool)
            n961 = Or(x=w1603, y=w1602) -> (x .or. y?=w1597:bool)
            n962 = case shown="True" w1597 {
              frame False {
              }
              frame True {
                n963 = local read "referenciaDisco"() -> (w1607:refnum<vi>)
                n964 = local read "coordenadas del mouse"() -> (w1606:T2)
                n965 = property class="Bool (strict)"(reference=w1607) -> (reference out=w1610:refnum<vi>, "Bounds"=w1608:T3)  [unwired: 1 in, 1 out]
                n966 = Divide(x=w1608, y=T3 {"Width"=2, "Height"=2}) -> (x/y=w1605:cluster{"Width":dbl, "Height":dbl})
                n967 = Subtract(x=w1606, y=w1605) -> (x-y=w1609:cluster{dbl, dbl})
                n968 = property class="Bool (strict)"(reference=w1610, "Position"=w1609) -> ()  [unwired: 1 in, 2 out]
              }
            }
          }
          frame 19 {
            # "Estado 19"
            # "Disco"
            # "Disco"
            n969 = local read "referenciaDisco"() -> (w1614:refnum<vi>)
            n970 = property class="Bool (strict)"(reference=w1614) -> ("Label.Text"=w1615:string)  [unwired: 1 in, 2 out]
            n971 = Equal?(x=w1615, y="1") -> (x = y?=w1617:bool)
            n972 = Equal?(x=w1615, y="2") -> (x = y?=w1616:bool)
            n973 = Or(x=w1617, y=w1616) -> (x .or. y?=w1611:bool)
            n974 = case shown="True" w1611 {
              frame False {
              }
              frame True {
                n975 = local read "referenciaDisco"() -> (w1621:refnum<vi>)
                n976 = local read "coordenadas del mouse"() -> (w1620:T2)
                n977 = property class="Bool (strict)"(reference=w1621) -> (reference out=w1624:refnum<vi>, "Bounds"=w1622:T3)  [unwired: 1 in, 1 out]
                n978 = Divide(x=w1622, y=T3 {"Width"=2, "Height"=2}) -> (x/y=w1619:cluster{"Width":dbl, "Height":dbl})
                n979 = Subtract(x=w1620, y=w1619) -> (x-y=w1623:cluster{dbl, dbl})
                n980 = property class="Bool (strict)"(reference=w1624, "Position"=w1623) -> ()  [unwired: 1 in, 2 out]
              }
            }
          }
          frame 20 {
            # "Estado 20"
            # "Disco"
            # "Disco"
            n981 = local read "referenciaDisco"() -> (w1628:refnum<vi>)
            n982 = property class="Bool (strict)"(reference=w1628) -> ("Label.Text"=w1629:string)  [unwired: 1 in, 2 out]
            n983 = Equal?(x=w1629, y="1") -> (x = y?=w1631:bool)
            n984 = Equal?(x=w1629, y="1") -> (x = y?=w1630:bool)
            n985 = Or(x=w1631, y=w1630) -> (x .or. y?=w1625:bool)
            n986 = case shown="True" w1625 {
              frame False {
              }
              frame True {
                n987 = local read "referenciaDisco"() -> (w1635:refnum<vi>)
                n988 = local read "coordenadas del mouse"() -> (w1634:T2)
                n989 = property class="Bool (strict)"(reference=w1635) -> (reference out=w1638:refnum<vi>, "Bounds"=w1636:T3)  [unwired: 1 in, 1 out]
                n990 = Divide(x=w1636, y=T3 {"Width"=2, "Height"=2}) -> (x/y=w1633:cluster{"Width":dbl, "Height":dbl})
                n991 = Subtract(x=w1634, y=w1633) -> (x-y=w1637:cluster{dbl, dbl})
                n992 = property class="Bool (strict)"(reference=w1638, "Position"=w1637) -> ()  [unwired: 1 in, 2 out]
              }
            }
          }
          frame 21 {
            # "Estado 21"
            # "Disco"
            # "Disco"
            n993 = local read "referenciaDisco"() -> (w1642:refnum<vi>)
            n994 = property class="Bool (strict)"(reference=w1642) -> ("Label.Text"=w1643:string)  [unwired: 1 in, 2 out]
            n995 = Equal?(x=w1643, y="1") -> (x = y?=w1645:bool)
            n996 = Equal?(x=w1643, y="2") -> (x = y?=w1644:bool)
            n997 = Or(x=w1645, y=w1644) -> (x .or. y?=w1639:bool)
            n998 = case shown="True" w1639 {
              frame False {
              }
              frame True {
                n999 = local read "referenciaDisco"() -> (w1649:refnum<vi>)
                n1000 = local read "coordenadas del mouse"() -> (w1648:T2)
                n1001 = property class="Bool (strict)"(reference=w1649) -> (reference out=w1652:refnum<vi>, "Bounds"=w1650:T3)  [unwired: 1 in, 1 out]
                n1002 = Divide(x=w1650, y=T3 {"Width"=2, "Height"=2}) -> (x/y=w1647:cluster{"Width":dbl, "Height":dbl})
                n1003 = Subtract(x=w1648, y=w1647) -> (x-y=w1651:cluster{dbl, dbl})
                n1004 = property class="Bool (strict)"(reference=w1652, "Position"=w1651) -> ()  [unwired: 1 in, 2 out]
              }
            }
          }
          frame 22 {
            # "Estado 22"
            # "Disco"
            # "Disco"
            n1005 = local read "referenciaDisco"() -> (w1656:refnum<vi>)
            n1006 = property class="Bool (strict)"(reference=w1656) -> ("Label.Text"=w1657:string)  [unwired: 1 in, 2 out]
            n1007 = Equal?(x=w1657, y="1") -> (x = y?=w1659:bool)
            n1008 = Equal?(x=w1657, y="3") -> (x = y?=w1658:bool)
            n1009 = Or(x=w1659, y=w1658) -> (x .or. y?=w1653:bool)
            n1010 = case shown="True" w1653 {
              frame False {
              }
              frame True {
                n1011 = local read "referenciaDisco"() -> (w1663:refnum<vi>)
                n1012 = local read "coordenadas del mouse"() -> (w1662:T2)
                n1013 = property class="Bool (strict)"(reference=w1663) -> (reference out=w1666:refnum<vi>, "Bounds"=w1664:T3)  [unwired: 1 in, 1 out]
                n1014 = Divide(x=w1664, y=T3 {"Width"=2, "Height"=2}) -> (x/y=w1661:cluster{"Width":dbl, "Height":dbl})
                n1015 = Subtract(x=w1662, y=w1661) -> (x-y=w1665:cluster{dbl, dbl})
                n1016 = property class="Bool (strict)"(reference=w1666, "Position"=w1665) -> ()  [unwired: 1 in, 2 out]
              }
            }
          }
          frame 23 {
            # "Estado 23"
            # "Disco"
            # "Disco"
            n1017 = local read "referenciaDisco"() -> (w1670:refnum<vi>)
            n1018 = property class="Bool (strict)"(reference=w1670) -> ("Label.Text"=w1671:string)  [unwired: 1 in, 2 out]
            n1019 = Equal?(x=w1671, y="1") -> (x = y?=w1673:bool)
            n1020 = Equal?(x=w1671, y="2") -> (x = y?=w1672:bool)
            n1021 = Or(x=w1673, y=w1672) -> (x .or. y?=w1667:bool)
            n1022 = case shown="True" w1667 {
              frame False {
              }
              frame True {
                n1023 = local read "referenciaDisco"() -> (w1677:refnum<vi>)
                n1024 = local read "coordenadas del mouse"() -> (w1676:T2)
                n1025 = property class="Bool (strict)"(reference=w1677) -> (reference out=w1680:refnum<vi>, "Bounds"=w1678:T3)  [unwired: 1 in, 1 out]
                n1026 = Divide(x=w1678, y=T3 {"Width"=2, "Height"=2}) -> (x/y=w1675:cluster{"Width":dbl, "Height":dbl})
                n1027 = Subtract(x=w1676, y=w1675) -> (x-y=w1679:cluster{dbl, dbl})
                n1028 = property class="Bool (strict)"(reference=w1680, "Position"=w1679) -> ()  [unwired: 1 in, 2 out]
              }
            }
          }
          frame 24 {
            # "Estado 24"
            # "Disco"
            # "Disco"
            n1029 = local read "referenciaDisco"() -> (w1684:refnum<vi>)
            n1030 = property class="Bool (strict)"(reference=w1684) -> ("Label.Text"=w1685:string)  [unwired: 1 in, 2 out]
            n1031 = Equal?(x=w1685, y="1") -> (x = y?=w1687:bool)
            n1032 = Equal?(x=w1685, y="2") -> (x = y?=w1686:bool)
            n1033 = Or(x=w1687, y=w1686) -> (x .or. y?=w1681:bool)
            n1034 = case shown="True" w1681 {
              frame False {
              }
              frame True {
                n1035 = local read "referenciaDisco"() -> (w1691:refnum<vi>)
                n1036 = local read "coordenadas del mouse"() -> (w1690:T2)
                n1037 = property class="Bool (strict)"(reference=w1691) -> (reference out=w1694:refnum<vi>, "Bounds"=w1692:T3)  [unwired: 1 in, 1 out]
                n1038 = Divide(x=w1692, y=T3 {"Width"=2, "Height"=2}) -> (x/y=w1689:cluster{"Width":dbl, "Height":dbl})
                n1039 = Subtract(x=w1690, y=w1689) -> (x-y=w1693:cluster{dbl, dbl})
                n1040 = property class="Bool (strict)"(reference=w1694, "Position"=w1693) -> ()  [unwired: 1 in, 2 out]
              }
            }
          }
          frame 25 {
            # "Estado 25"
            # "Disco"
            # "Disco"
            n1041 = local read "referenciaDisco"() -> (w1698:refnum<vi>)
            n1042 = property class="Bool (strict)"(reference=w1698) -> ("Label.Text"=w1699:string)  [unwired: 1 in, 2 out]
            n1043 = Equal?(x=w1699, y="1") -> (x = y?=w1701:bool)
            n1044 = Equal?(x=w1699, y="1") -> (x = y?=w1700:bool)
            n1045 = Or(x=w1701, y=w1700) -> (x .or. y?=w1695:bool)
            n1046 = case shown="True" w1695 {
              frame False {
              }
              frame True {
                n1047 = local read "referenciaDisco"() -> (w1705:refnum<vi>)
                n1048 = local read "coordenadas del mouse"() -> (w1704:T2)
                n1049 = property class="Bool (strict)"(reference=w1705) -> (reference out=w1708:refnum<vi>, "Bounds"=w1706:T3)  [unwired: 1 in, 1 out]
                n1050 = Divide(x=w1706, y=T3 {"Width"=2, "Height"=2}) -> (x/y=w1703:cluster{"Width":dbl, "Height":dbl})
                n1051 = Subtract(x=w1704, y=w1703) -> (x-y=w1707:cluster{dbl, dbl})
                n1052 = property class="Bool (strict)"(reference=w1708, "Position"=w1707) -> ()  [unwired: 1 in, 2 out]
              }
            }
          }
          frame 26 {
            # "Estado 26"
            # "Disco"
            # "Disco"
            n1053 = local read "referenciaDisco"() -> (w1712:refnum<vi>)
            n1054 = property class="Bool (strict)"(reference=w1712) -> ("Label.Text"=w1713:string)  [unwired: 1 in, 2 out]
            n1055 = Equal?(x=w1713, y="1") -> (x = y?=w1715:bool)
            n1056 = Equal?(x=w1713, y="3") -> (x = y?=w1714:bool)
            n1057 = Or(x=w1715, y=w1714) -> (x .or. y?=w1709:bool)
            n1058 = case shown="True" w1709 {
              frame False {
              }
              frame True {
                n1059 = local read "referenciaDisco"() -> (w1719:refnum<vi>)
                n1060 = local read "coordenadas del mouse"() -> (w1718:T2)
                n1061 = property class="Bool (strict)"(reference=w1719) -> (reference out=w1722:refnum<vi>, "Bounds"=w1720:T3)  [unwired: 1 in, 1 out]
                n1062 = Divide(x=w1720, y=T3 {"Width"=2, "Height"=2}) -> (x/y=w1717:cluster{"Width":dbl, "Height":dbl})
                n1063 = Subtract(x=w1718, y=w1717) -> (x-y=w1721:cluster{dbl, dbl})
                n1064 = property class="Bool (strict)"(reference=w1722, "Position"=w1721) -> ()  [unwired: 1 in, 2 out]
              }
            }
          }
          frame 27 {
            # "Estado 26"
            # "Disco"
            # "Disco"
            n1065 = local read "referenciaDisco"() -> (w1726:refnum<vi>)
            n1066 = property class="Bool (strict)"(reference=w1726) -> ("Label.Text"=w1727:string)  [unwired: 1 in, 2 out]
            n1067 = Equal?(x=w1727, y="1") -> (x = y?=w1729:bool)
            n1068 = Equal?(x=w1727, y="2") -> (x = y?=w1728:bool)
            n1069 = Or(x=w1729, y=w1728) -> (x .or. y?=w1723:bool)
            n1070 = case shown="True" w1723 {
              frame False {
              }
              frame True {
                n1071 = local read "referenciaDisco"() -> (w1733:refnum<vi>)
                n1072 = local read "coordenadas del mouse"() -> (w1732:T2)
                n1073 = property class="Bool (strict)"(reference=w1733) -> (reference out=w1736:refnum<vi>, "Bounds"=w1734:T3)  [unwired: 1 in, 1 out]
                n1074 = Divide(x=w1734, y=T3 {"Width"=2, "Height"=2}) -> (x/y=w1731:cluster{"Width":dbl, "Height":dbl})
                n1075 = Subtract(x=w1732, y=w1731) -> (x-y=w1735:cluster{dbl, dbl})
                n1076 = property class="Bool (strict)"(reference=w1736, "Position"=w1735) -> ()  [unwired: 1 in, 2 out]
              }
            }
          }
        }
      }
    }
  }
  n1077 = while {
    stop <- FALSE stop-if-true
    # "Eventos principales"
    n1078 = event shown="[4] \"1\", \"2\", \"3\", \"4\", \"5\": Mouse Down" {
      selector: _ -> [_ _ _ _ _]
      dyn-events: _ -> [_ _ _ _ _]
      timeout: 10 -> [_ _ _ _ _]
      event Timeout {
        n1079 = event-data() -> ()  [unwired: 1 in, 3 out]
        n1080 = local read "estado"() -> (w1743:u16)
        n1081 = Equal?(x=w1743, y=u16 25) -> (x = y?=w1741:bool)
        n1082 = local read "Numero de discos"() -> (w1740:enum16{"3", "4", "5"})
        n1083 = property on="mensaje" class="Str"("Visible"=w1741) -> ()  [unwired: 2 in, 2 out]
        n1084 = case shown="True" w1741 {
          frame False {
          }
          frame True {
            n1085 = local read "Tu numero de movimientos"() -> (w1752:i16)
            n1086 = Equal?(x=w1752, y=i16 7) -> (x = y?=w1750:bool)
            n1087 = Select(t="Game Over !!!\nFelicidades! Lo has conseguido en 7 movimientos.", s=w1750, f="Game Over !!!\nMuy bien, lo has conseguido pero puedes mejorar.") -> (s? t:f=→"mensaje":string)
          }
        }
        n1088 = case shown="\"5\"" w1740 {
          tunnel: ["Paso 01: Pasar disco 1 de la torre 1 a la torre 3.\nPaso 02: Pasar disco 2 de la torre 1 a la torre 2.\nPaso 03: Pasar disco 1 de la torre 3 a la torre 2.\nPaso 04: Pasar disco 3 de la torre 1 a la torre 3.\nPaso 05: Pasar disco 1 de la torre 2 a la torre 1.\nPaso 06: Pasar disco 2 de la torre 2 a la torre 3.\nPaso 07: Pasar disco 1 de la torre 1 a la torre 3." "Paso 01: Pasar disco 1 de la torre 1 a la torre 2.\nPaso 02: Pasar disco 2 de la torre 1 a la torre 3.\nPaso 03: Pasar disco 1 de la torre 2 a la torre 3.\nPaso 04: Pasar disco 3 de la torre 1 a la torre 2.\nPaso 05: Pasar disco 1 de la torre 3 a la torre 1.\nPaso 06: Pasar disco 2 de la torre 3 a la torre 2.\nPaso 07: Pasar disco 1 de la torre 1 a la torre 2.\nPaso 08: Pasar disco 4 de la torre 1 a la torre 3.\nPaso 09: Pasar disco 1 de la torre 2 a la torre 3.\nPaso 10: Pasar disco 2 de la torre 2 a la torre 1.\nPaso 11: Pasar disco 1 de la torre 3 a la torre 1.\nPaso 12: Pasar disco 3 de la torre 2 a la torre 3.\nPaso 13: Pasar disco 1 de la torre 1 a la torre 2.\nPaso 14: Pasar disco 2 de la torre 1 a la torre 3.\nPaso 15: Pasar disco 1 de la torre 2 a la torre 3." ""] -> w1739
          frame "3", Default {
          }
          frame "4" {
          }
          frame "5" {
          }
        }
        "pasos" <- w1739
      }
      event "Numero de discos": Value Change {
        n1089 = event-data() -> ("CtlRef"=w1754:refnum<vi>, "OldVal"=w1753:enum16{"3", "4", "5"})  [unwired: 1 in, 4 out]
        n1090 = property class="Enum (strict)"(reference=w1754) -> ("Value"=w1757:enum16{"3", "4", "5"})  [unwired: 1 in, 2 out]
        n1091 = Two Button Dialog(message="El juego actual se cancelará, ¿te gustaría continuar?") -> (T button?=w1755:bool)  [unwired: 2 in]
        n1092 = case shown="True" w1755 {
          tunnel: w1757 -> [_ w1762]
          tunnel: w1754 -> [_ _]
          tunnel: w1753 -> [w1758 _]
          frame False {
            n1093 = local write "Numero de discos"(w1758) -> ()
          }
          frame True {
            n1094 = case shown="\"4\"" w1762 {
              tunnel: [u16 7 ("Minimos de movimientos") u16 15 ("Minimos de movimientos") u16 31 ("Minimos de movimientos")] -> w1761
              frame "3", Default {
                n1095 = property on="3" class="Bool (strict)"("Position"=T1 {"Left"=163, "Top"=653}) -> ()  [unwired: 2 in, 2 out]
                n1096 = property on="4" class="Bool (strict)"("Position"=T1 {"Left"=133, "Top"=1000}) -> ()  [unwired: 2 in, 2 out]
                n1097 = property on="5" class="Bool (strict)"("Position"=T1 {"Left"=103, "Top"=1000}) -> ()  [unwired: 2 in, 2 out]
                n1098 = property on="1" class="Bool (strict)"("Position"=T1 {"Left"=223, "Top"=541}) -> ()  [unwired: 2 in, 2 out]
                n1099 = property on="2" class="Bool (strict)"("Position"=T1 {"Left"=193, "Top"=597}) -> ()  [unwired: 2 in, 2 out]
                n1100 = property on="3" class="Bool (strict)"("Visible"=TRUE) -> ()  [unwired: 2 in, 2 out]
                n1101 = property on="4" class="Bool (strict)"("Visible"=FALSE) -> ()  [unwired: 2 in, 2 out]
                n1102 = property on="5" class="Bool (strict)"("Visible"=FALSE) -> ()  [unwired: 2 in, 2 out]
                n1103 = property on="1" class="Bool (strict)"("Visible"=TRUE) -> ()  [unwired: 2 in, 2 out]
                n1104 = property on="2" class="Bool (strict)"("Visible"=TRUE) -> ()  [unwired: 2 in, 2 out]
              }
              frame "4" {
                n1105 = property on="3" class="Bool (strict)"("Position"=T1 {"Left"=163, "Top"=597}) -> ()  [unwired: 2 in, 2 out]
                n1106 = property on="4" class="Bool (strict)"("Position"=T1 {"Left"=133, "Top"=653}) -> ()  [unwired: 2 in, 2 out]
                n1107 = property on="5" class="Bool (strict)"("Position"=T1 {"Left"=103, "Top"=1000}) -> ()  [unwired: 2 in, 2 out]
                n1108 = property on="1" class="Bool (strict)"("Position"=T1 {"Left"=223, "Top"=485}) -> ()  [unwired: 2 in, 2 out]
                n1109 = property on="2" class="Bool (strict)"("Position"=T1 {"Left"=193, "Top"=541}) -> ()  [unwired: 2 in, 2 out]
                n1110 = property on="3" class="Bool (strict)"("Visible"=TRUE) -> ()  [unwired: 2 in, 2 out]
                n1111 = property on="4" class="Bool (strict)"("Visible"=TRUE) -> ()  [unwired: 2 in, 2 out]
                n1112 = property on="5" class="Bool (strict)"("Visible"=FALSE) -> ()  [unwired: 2 in, 2 out]
                n1113 = property on="1" class="Bool (strict)"("Visible"=TRUE) -> ()  [unwired: 2 in, 2 out]
                n1114 = property on="2" class="Bool (strict)"("Visible"=TRUE) -> ()  [unwired: 2 in, 2 out]
              }
              frame "5" {
                n1115 = property on="3" class="Bool (strict)"("Position"=T1 {"Left"=163, "Top"=541}) -> ()  [unwired: 2 in, 2 out]
                n1116 = property on="4" class="Bool (strict)"("Position"=T1 {"Left"=133, "Top"=597}) -> ()  [unwired: 2 in, 2 out]
                n1117 = property on="5" class="Bool (strict)"("Position"=T1 {"Left"=103, "Top"=653}) -> ()  [unwired: 2 in, 2 out]
                n1118 = property on="1" class="Bool (strict)"("Position"=T1 {"Left"=223, "Top"=429}) -> ()  [unwired: 2 in, 2 out]
                n1119 = property on="2" class="Bool (strict)"("Position"=T1 {"Left"=193, "Top"=485}) -> ()  [unwired: 2 in, 2 out]
                n1120 = property on="3" class="Bool (strict)"("Visible"=TRUE) -> ()  [unwired: 2 in, 2 out]
                n1121 = property on="4" class="Bool (strict)"("Visible"=TRUE) -> ()  [unwired: 2 in, 2 out]
                n1122 = property on="5" class="Bool (strict)"("Visible"=TRUE) -> ()  [unwired: 2 in, 2 out]
                n1123 = property on="1" class="Bool (strict)"("Visible"=TRUE) -> ()  [unwired: 2 in, 2 out]
                n1124 = property on="2" class="Bool (strict)"("Visible"=TRUE) -> ()  [unwired: 2 in, 2 out]
              }
            }
            n1125 = local write "Tu numero de movimientos"(i16 0 ("Tu numero de movimientos")) -> ()
            n1126 = local write "Minimos de movimientos"(w1761) -> ()
            n1127 = local write "estado"(u16 0 ("estado")) -> ()
          }
        }
      }
      event "Iniciar": Mouse Down {
        n1128 = event-data() -> ()  [unwired: 1 in, 8 out]
        n1129 = local read "Numero de discos"() -> (w1796:enum16{"3", "4", "5"})
        n1130 = Two Button Dialog(message="El juego actual se cancelará, ¿te gustaría continuar?") -> (T button?=w1798:bool)  [unwired: 2 in]
        n1131 = case shown="False" w1798 {
          tunnel: w1796 -> [_ w1802]
          frame False {
          }
          frame True {
            n1132 = case shown="\"3\", Default" w1802 {
              tunnel: [u16 7 ("Minimos de movimientos") u16 15 ("Minimos de movimientos") u16 31 ("Minimos de movimientos")] -> w1801
              frame "3", Default {
                n1133 = property on="3" class="Bool (strict)"("Position"=T1 {"Left"=163, "Top"=653}) -> ()  [unwired: 2 in, 2 out]
                n1134 = property on="4" class="Bool (strict)"("Position"=T1 {"Left"=133, "Top"=1000}) -> ()  [unwired: 2 in, 2 out]
                n1135 = property on="5" class="Bool (strict)"("Position"=T1 {"Left"=103, "Top"=1000}) -> ()  [unwired: 2 in, 2 out]
                n1136 = property on="1" class="Bool (strict)"("Position"=T1 {"Left"=223, "Top"=541}) -> ()  [unwired: 2 in, 2 out]
                n1137 = property on="2" class="Bool (strict)"("Position"=T1 {"Left"=193, "Top"=597}) -> ()  [unwired: 2 in, 2 out]
                n1138 = property on="3" class="Bool (strict)"("Visible"=TRUE) -> ()  [unwired: 2 in, 2 out]
                n1139 = property on="4" class="Bool (strict)"("Visible"=FALSE) -> ()  [unwired: 2 in, 2 out]
                n1140 = property on="5" class="Bool (strict)"("Visible"=FALSE) -> ()  [unwired: 2 in, 2 out]
                n1141 = property on="1" class="Bool (strict)"("Visible"=TRUE) -> ()  [unwired: 2 in, 2 out]
                n1142 = property on="2" class="Bool (strict)"("Visible"=TRUE) -> ()  [unwired: 2 in, 2 out]
              }
              frame "4" {
                # "653"
                # "597"
                # "541"
                # "485"
                # "429"
                n1143 = property on="3" class="Bool (strict)"("Position"=T1 {"Left"=163, "Top"=597}) -> ()  [unwired: 2 in, 2 out]
                n1144 = property on="4" class="Bool (strict)"("Position"=T1 {"Left"=133, "Top"=653}) -> ()  [unwired: 2 in, 2 out]
                n1145 = property on="5" class="Bool (strict)"("Position"=T1 {"Left"=103, "Top"=1000}) -> ()  [unwired: 2 in, 2 out]
                n1146 = property on="1" class="Bool (strict)"("Position"=T1 {"Left"=223, "Top"=485}) -> ()  [unwired: 2 in, 2 out]
                n1147 = property on="2" class="Bool (strict)"("Position"=T1 {"Left"=193, "Top"=541}) -> ()  [unwired: 2 in, 2 out]
                n1148 = property on="3" class="Bool (strict)"("Visible"=TRUE) -> ()  [unwired: 2 in, 2 out]
                n1149 = property on="4" class="Bool (strict)"("Visible"=TRUE) -> ()  [unwired: 2 in, 2 out]
                n1150 = property on="5" class="Bool (strict)"("Visible"=FALSE) -> ()  [unwired: 2 in, 2 out]
                n1151 = property on="1" class="Bool (strict)"("Visible"=TRUE) -> ()  [unwired: 2 in, 2 out]
                n1152 = property on="2" class="Bool (strict)"("Visible"=TRUE) -> ()  [unwired: 2 in, 2 out]
              }
              frame "5" {
                n1153 = property on="3" class="Bool (strict)"("Position"=T1 {"Left"=163, "Top"=541}) -> ()  [unwired: 2 in, 2 out]
                n1154 = property on="4" class="Bool (strict)"("Position"=T1 {"Left"=133, "Top"=597}) -> ()  [unwired: 2 in, 2 out]
                n1155 = property on="5" class="Bool (strict)"("Position"=T1 {"Left"=103, "Top"=653}) -> ()  [unwired: 2 in, 2 out]
                n1156 = property on="1" class="Bool (strict)"("Position"=T1 {"Left"=223, "Top"=429}) -> ()  [unwired: 2 in, 2 out]
                n1157 = property on="2" class="Bool (strict)"("Position"=T1 {"Left"=193, "Top"=485}) -> ()  [unwired: 2 in, 2 out]
                n1158 = property on="3" class="Bool (strict)"("Visible"=TRUE) -> ()  [unwired: 2 in, 2 out]
                n1159 = property on="4" class="Bool (strict)"("Visible"=TRUE) -> ()  [unwired: 2 in, 2 out]
                n1160 = property on="5" class="Bool (strict)"("Visible"=TRUE) -> ()  [unwired: 2 in, 2 out]
                n1161 = property on="1" class="Bool (strict)"("Visible"=TRUE) -> ()  [unwired: 2 in, 2 out]
                n1162 = property on="2" class="Bool (strict)"("Visible"=TRUE) -> ()  [unwired: 2 in, 2 out]
              }
            }
            n1163 = local write "Tu numero de movimientos"(i16 0 ("Tu numero de movimientos")) -> ()
            n1164 = local write "Minimos de movimientos"(w1801) -> ()
            n1165 = local write "estado"(u16 0 ("estado")) -> ()
          }
        }
      }
      event "instrucciones": Mouse Down {
        n1166 = event-data() -> ()  [unwired: 1 in, 8 out]
        n1167 = property on="pasos" class="Str"() -> ("Visible"=w1837:bool)  [unwired: 2 in, 2 out]
        n1168 = Not(x=w1837) -> (.not. x?=w1836:bool)
        n1169 = property on="pasos" class="Str"("Visible"=w1836) -> ()  [unwired: 2 in, 2 out]
      }
      event "1", "2", "3", "4", "5": Mouse Down {
        # "Left == horizontal\nTop == vertical"
        # "Torre1\nRango horizontal\n70 - 570\nRango vertical\n210 - 710\n\n\nTorre2\nRango horizontal\n610 - 1115\nRango vertical\n210 - 710\n\n\nTorre2\nRango horizontal\n1150 - 1650\nRango vertical\n210 - 710"
        n1170 = event-data() -> ("CtlRef"=w1840:refnum<vi>)  [unwired: 1 in]
        "referenciaDisco" <- w1840
        n1171 = property class="Bool (strict)"(reference=w1840) -> ("Position"=→"positionIncialDisco":T1, "Label.Text"=→"discoaMover":string)  [unwired: 1 in, 2 out]
        n1172 = local read "coordenadas del mouse"() -> (w1839:T2)
        n1173 = call "Q2_validar torre.vi"("coordenadas del mouse"=w1839) -> ("Torre"=w1838:i32)  [unwired: 3 in, 3 out]
        n1174 = local write "positionIncialTorre"(w1838) -> ()
        "mouseActivoPorEvento?" <- TRUE ("mouseActivo?")
      }
    }
  }
  n1175 = while {
    stop <- FALSE stop-if-true
    # "Evento para leer posicion del mouse"
    n1176 = event shown="[1] \"Pane\": Mouse Move" {
      selector: _ -> [_ _]
      dyn-events: _ -> [_ _]
      timeout: _ -> [_ _]
      event Timeout {
        n1177 = event-data() -> ()  [unwired: 1 in, 1 out]
      }
      event Mouse Move {
        n1178 = event-data() -> ("Coords"=→"coordenadas del mouse":T2)  [unwired: 1 in]
      }
    }
  }
  n1179 = call-poly <vilib>:"Close Input Device.vi"("error in (no error)"=w3, "device ID"=w4) -> ()  [unwired: 8 in, 1 out]
  "1" <- TRUE ("disco1")
  "2" <- TRUE ("disco2")
  "3" <- TRUE ("disco3")
  "4" <- TRUE ("disco4")
  "5" <- TRUE ("disco5")
  "TORRE1" <- TRUE ("TORRE1")
  "TORRE2" <- TRUE ("TORRE2")
  "TORRE3" <- TRUE ("TORRE3")
  "BASE" <- TRUE ("BASE")
  "positionIncialTorre" <- 1 ("positionIncialTorre")
  "estado" <- u16 0 ("estado")
  "mouse" <- FALSE ("mouse")
  "evento" <- u32 0 ("evento")
